vi "MAIN - PECT - Autonics.vi"() -> ()   [LabVIEW 2018]
uses:
  Control 1.ctl
  <vilib>/DAQmx/write.llb/DAQmx Write (Analog 1D Wfm NChan NSamp).vi
  <vilib>/DAQmx/read.llb/DAQmx Read (Analog 1D Wfm NChan NSamp).vi
  <vilib>/Instr/_visa.llb/VISA Configure Serial Port (Instr).vi
  <vilib>/DAQmx/create/channels.llb/DAQmx Create Channel (AI-Voltage-Basic).vi
  <vilib>/DAQmx/configure/timing.llb/DAQmx Timing (Sample Clock).vi
  <vilib>/DAQmx/configure/trigger.llb/DAQmx Start Trigger (Digital Edge).vi
  <vilib>/DAQmx/create/channels.llb/DAQmx Create Channel (AO-Voltage-Basic).vi
  <vilib>/DAQmx/miscellaneous.llb/DAQmx Fill In Error Info.vi
  Global_data.vi
  <vilib>/express/express analysis/Spectral/Block/exnSpectralBlock spectral measurements PSD poly.vi
  <vilib>/express/express analysis/Spectral/Block/exnSpectralBlock spectral measurements PSD WFM.vi
  <vilib>/express/express analysis/Spectral/XNode/ExpressSpectralMeasurementsBlockNode.xnode
  <resource>/objmgr/daqmx.rc
  <vilib>/measure/NI_MABase.lvlib
  <vilib>/Platform/NI_3dgraph.lvlib
  <vilib>/DAQmx/read.llb/DAQmx Read (Counter U32 1Chan 1Samp).vi
  <vilib>/DAQmx/create/channels.llb/DAQmx Create Channel (CI-Count Edges).vi
panel:
  out "dy":dbl[][](array[numeric])
  in  "2D Array In":dbl[][](array[numeric])
  out "Output":dbl[][](array[numeric])
  out "Current  Position (mm)":dbl=34.0
  out "Acquire":bool
  out "Numeric":dbl=34.0
  out "Enum":T1(ring)
  in  "Direction (+)":string="+"
  in  "Tab Control 3":enum32{"Control", "Data Processing"}(tab)
  in  "Home":bool
  in  "Exit":bool
  in  "Scan":bool
  in  "Move Dis(mm)":dbl=180.0
  in  "Right":bool
  in  "Forward":bool
  in  "Left":bool
  in  "Backward":bool
  in  "Stop":bool
  in  "Duty cycle %":dbl=50.0 format="%#.2f"
  in  "Pulser Trigger":tag="/Dev3/PFI0"
  in  "Edge":i32(ring)=10280 items=["Rising"=10280, "Falling"=10171]
  in  "2 Plots":bool
  in  "Offset":bool
  in  "Open csv":bool
  in  "Save Scan mode":bool caption="Save Process"
  in  "Gate 1":dbl
  in  "Gate 2":dbl=50.0
  in  "Pulse generator":T3={"Waveform Type"=2, "Amplitude"=2.0, "Frequency"=300.0} {"Frequency" format="%0.2p"; "Amplitude" format="%0.2p"; "Waveform Type" items=["Sine Wave", "Triangle Wave", "Square Wave", "Sawtooth Wave"]}
  in  "Open tdms":bool
  in  "Motor Counter Terminal":tag="PFI8"
  in  "Motor counter":tag="Dev6/ctr0"
  out "Motor Pulse Count":i32
  in  "Cursor":bool=TRUE
  in  "Repair Line Col":bool
  in  "Repair Line Row":bool
  in  "Line Col":dbl=167.0
  in  "Line Row":dbl
  in  "Y-max":dbl
  in  "Y-min":dbl
  in  "X-max":dbl
  in  "X-min":dbl
  in  "Inverse":bool caption="Scan"
  in  "ViewMode":i32(ring) items=["cwViewXYPlane", "cwViewXZPlane", "cwViewYZPlane", "cwViewUserDefined"]
  in  "Plot style":i32(ring)=5 items=["cwLine"=1, "cwPoint"=2, "cwLinePoint"=3, "cwHiddenLine"=4, "cwSurface"=5, "cwSurfaceLine"=6, "cwSurfaceNormal"=7, "cwContourLine"=8, "cwSurfaceContour"=9]
  in  "ColorMapAutoScale":bool=TRUE
  in  "Max":dbl=0.6
  in  "Min":dbl=-0.8
  in  "low cutoff freq: fl":dbl=40.0 format="%0.2f"
  in  "Filter":bool caption="Scan"
  in  "Backindex":i32
  in  "Backdata":bool caption="Scan"
  in  "Odd":bool caption="Scan"
  in  "DiffX":bool caption="Scan"
  in  "DiffY":bool caption="Scan"
  in  "Abs":bool caption="Scan"
  in  "Trim data":bool caption="Scan"
  in  "Return":bool caption="Scan"
  out "No.data":i32=160450
  in  "Tab Control 2":T4(tab)=enum."Lift-Off"
  out "Hall sensors signal":waveform(dbl)[](graph)=[{"t0"=timestamp(3764892578.4882636 s since 1904-01-01), "dt"=9.999999999999972e-06, "Y"=array[333 elements], "attributes"=variant("NI_ChannelName"=variant(string "Acquisition Task0"), "NI_UnitDescription"=variant(string "Volts"))}, {"t0"=timestamp(3764892578.4882636 s since 1904-01-01), "dt"=9.999999999999972e-06, "Y"=array[333 elements], "attributes"=variant("NI_ChannelName"=variant(string "Acquisition Task0"), "NI_UnitDescription"=variant(string "Volts"))}]
  out "Feature Extraction":dbl(graph)=2.323572486727786
  out "Power spectral density":cluster{"f0":dbl, "df":dbl, "magnitude":dbl[]}[](graph)=[{"f0"=0.0, "df"=300.30030030030116, "magnitude"=[-36.20180290677153, -20.90483721068611, -24.582468351224577, -31.42004868416134, -34.14223622321665, -37.70031787769031, -39.88091390016968, -42.570527872297575, -44.447142301932836, -46.690350484337216, -48.33027794655095, -50.25956499863859, -51.72550449795308, -53.39972065859007, -54.70440561731976, -56.21393447819807, -57.42147971089571, -58.793048346684444, -59.91128808109209, -61.1290372398805, -62.12849722306457, -63.101740591151284, -63.85083396363265, -65.0208550120241, -66.15115529173912, -67.20106472607435, -68.15468936452316, -69.13750415748885, -69.85723332409452, -70.64087441700111, -71.384683910046, -72.10421787745543, -72.7097904698358, -73.76225860074786, -74.58656508865108, -75.0441981120336, -75.64428414686775, -76.36908179290627, -76.94177220206493, -77.59120517409957, -78.33715910390706, -79.06347610630218, -79.2988856080301, -79.948424760671, -80.92068806415895, -81.77260728293177, -81.8128457263302, -84.88880957913159, -83.99592011335217, -82.99389217923485, -86.3974807070411, -83.85611495905388, -85.04739834436776, -85.25536921781624, -86.04780288701166, -86.74967696173687, -87.4250358191504, -88.33981201247339, -88.29806177830426, -88.20989281176266, -90.52050898830177, -92.73295435458243, -91.05315268517512, -89.84986904119829, -90.1243991759323, -90.08140850500105, -90.51527924221807, -91.45597364465522, -92.37045984758105, -93.05963774586344, -93.27766487428342, -92.9148468037372, -93.45821417413453, -93.416885589902, -93.97004881358691, -100.16926286158659, -103.25126222782166, -97.916857786497, -97.02995967192803, -95.41315314455832, -85.28282838125556, -91.11753429616104, -98.34800147586265, -95.8173712278324, -95.84520134535146, -96.4411910777247, -97.79095251820118, -98.76337971056503, -99.52978551104567, -99.8473172312514, -99.7267196324173, -98.48034706548019, -98.4052682848681, -98.99036338133746, -99.81336358949763, -102.0234560078495, -106.30264837390989, -114.30404783446014, -110.5666525988822, -104.07428115468332, -106.56951387813052, -113.47776650834994, -104.8106680242567, -100.96454968097595, -103.26069189712638, -101.90020017156294, -97.35968680838327, -96.96723228272809, -104.78687680019844, -114.24669922913404, -105.47220635299163, -98.95153167883362, -95.72018168888859, -96.8791317080412, -103.59986254747135, -102.32961820827316, -103.50838559146095, -106.10294185717709, -107.56586317626123, -106.21980505741361, -106.75509409282448, -105.05473267043033, -105.72146157564094, -110.05572010167114, -103.09831905065673, -100.15680582227236, -106.62655602557932, -106.04738128978546, -102.29039381337167, -107.38407353728698, -106.04045858582134, -110.27062566191805, -101.58023602789737, -100.24058473092191, -101.82465844258417, -100.49593108832102, -107.37379008605268, -111.32932544252029, -113.33511250623216, -114.1358519115806, -116.77137581473383, -119.68802410059281, -122.30038665579934, -112.78569209435597, -113.20144887694318, -114.95593587471012, -114.2945515663458, -111.45765285754484, -108.98035354159111, -102.76141277040767, -94.76605415382379, -94.53014863989041, -102.82086347018918, -104.07676059492192, -93.56502067634786, -82.01368063028869, -82.14520649644004, -92.93791399449489, -115.13858185041988, -111.90044783845615, -102.8580225326784, -106.35532255950906, -109.47985188850006, -118.27062096579498, -133.54486345969963, -117.32910571092162, -119.97301996033957]}, {"f0"=0.0, "df"=300.30030030030116, "magnitude"=[-36.20180290677153, -20.90483721068611, -24.582468351224577, -31.42004868416134, -34.14223622321665, -37.70031787769031, -39.88091390016968, -42.570527872297575, -44.447142301932836, -46.690350484337216, -48.33027794655095, -50.25956499863859, -51.72550449795308, -53.39972065859007, -54.70440561731976, -56.21393447819807, -57.42147971089571, -58.793048346684444, -59.91128808109209, -61.1290372398805, -62.12849722306457, -63.101740591151284, -63.85083396363265, -65.0208550120241, -66.15115529173912, -67.20106472607435, -68.15468936452316, -69.13750415748885, -69.85723332409452, -70.64087441700111, -71.384683910046, -72.10421787745543, -72.7097904698358, -73.76225860074786, -74.58656508865108, -75.0441981120336, -75.64428414686775, -76.36908179290627, -76.94177220206493, -77.59120517409957, -78.33715910390706, -79.06347610630218, -79.2988856080301, -79.948424760671, -80.92068806415895, -81.77260728293177, -81.8128457263302, -84.88880957913159, -83.99592011335217, -82.99389217923485, -86.3974807070411, -83.85611495905388, -85.04739834436776, -85.25536921781624, -86.04780288701166, -86.74967696173687, -87.4250358191504, -88.33981201247339, -88.29806177830426, -88.20989281176266, -90.52050898830177, -92.73295435458243, -91.05315268517512, -89.84986904119829, -90.1243991759323, -90.08140850500105, -90.51527924221807, -91.45597364465522, -92.37045984758105, -93.05963774586344, -93.27766487428342, -92.9148468037372, -93.45821417413453, -93.416885589902, -93.97004881358691, -100.16926286158659, -103.25126222782166, -97.916857786497, -97.02995967192803, -95.41315314455832, -85.28282838125556, -91.11753429616104, -98.34800147586265, -95.8173712278324, -95.84520134535146, -96.4411910777247, -97.79095251820118, -98.76337971056503, -99.52978551104567, -99.8473172312514, -99.7267196324173, -98.48034706548019, -98.4052682848681, -98.99036338133746, -99.81336358949763, -102.0234560078495, -106.30264837390989, -114.30404783446014, -110.5666525988822, -104.07428115468332, -106.56951387813052, -113.47776650834994, -104.8106680242567, -100.96454968097595, -103.26069189712638, -101.90020017156294, -97.35968680838327, -96.96723228272809, -104.78687680019844, -114.24669922913404, -105.47220635299163, -98.95153167883362, -95.72018168888859, -96.8791317080412, -103.59986254747135, -102.32961820827316, -103.50838559146095, -106.10294185717709, -107.56586317626123, -106.21980505741361, -106.75509409282448, -105.05473267043033, -105.72146157564094, -110.05572010167114, -103.09831905065673, -100.15680582227236, -106.62655602557932, -106.04738128978546, -102.29039381337167, -107.38407353728698, -106.04045858582134, -110.27062566191805, -101.58023602789737, -100.24058473092191, -101.82465844258417, -100.49593108832102, -107.37379008605268, -111.32932544252029, -113.33511250623216, -114.1358519115806, -116.77137581473383, -119.68802410059281, -122.30038665579934, -112.78569209435597, -113.20144887694318, -114.95593587471012, -114.2945515663458, -111.45765285754484, -108.98035354159111, -102.76141277040767, -94.76605415382379, -94.53014863989041, -102.82086347018918, -104.07676059492192, -93.56502067634786, -82.01368063028869, -82.14520649644004, -92.93791399449489, -115.13858185041988, -111.90044783845615, -102.8580225326784, -106.35532255950906, -109.47985188850006, -118.27062096579498, -133.54486345969963, -117.32910571092162, -119.97301996033957]}]
  in  "Add LF":bool
  in  "Save LF":bool caption="Save Process"
  in  "3D Surface":refnum<k7>(container)
  out "Record path":path=path "F:/NDT PECT/MAIN/data/0404/PECT_default.tdms" caption="selected path"
  out "Feature extraction scan":dbl[](graph)=[1.5306579414004435, 1.5317305059894941, 1.5326200461021255, 1.5328476302606462, 1.5329951898783618, 1.5347077460020615, 1.5340483037518404, 1.538225484080516, 1.5384156334587897, 1.5342859972971667, 1.5376573962153353, 1.5346896305782285, 1.5333408499151915, 1.5374363281462833, 1.5365733968770157, 1.5371060772351082, 1.5377661752425886, 1.5331402955096363, 1.5333082171292225, 1.5328402076589231, 1.5319284519372456, 1.5339877687593646, 1.5306010503955654, 1.5307758007425079, 1.5329574004689674, 1.5329084504666064, 1.5321700113481294, 1.5313764189356205, 1.5320421800954864, 1.532745648807346, 1.5335423450461179, 1.5304344707607942, 1.5310324412127772, 0.0, 0.0, 0.0, 0.0, 0.0, 0.0, 0.0, 0.0, 0.0, 0.0, 0.0, 0.0, 0.0, 0.0, 0.0, 0.0, 0.0, 0.0, 0.0, 0.0, 0.0, 0.0, 0.0, 0.0, 0.0, 0.0, 0.0, 0.0, 0.0, 0.0, 0.0, 0.0, 0.0, 0.0, 0.0, 0.0, 0.0, 0.0, 0.0, 0.0, 0.0, 0.0, 0.0, 0.0, 0.0, 0.0, 0.0, 0.0, 0.0, 0.0, 0.0, 0.0, 0.0, 0.0, 0.0, 0.0, 0.0, 0.0, 0.0, 0.0, 0.0, 0.0, 0.0, 0.0, 0.0, 0.0, 0.0, 0.0, 0.0, 0.0, 0.0, 0.0, 0.0, 0.0, 0.0, 0.0, 0.0, 0.0, 0.0, 0.0, 0.0, 0.0, 0.0, 0.0, 0.0, 0.0, 0.0, 0.0, 0.0, 0.0, 0.0, 0.0, 0.0, 0.0, 0.0, 0.0, 0.0, 0.0, 0.0, 0.0, 0.0, 0.0, 0.0, 0.0, 0.0, 0.0, 0.0]
  in  "View Mode":bool caption="Scan"
  out "Hall sensors signal lf":dbl[][](graph)
  in  "Open":bool
  in  "Filter lf":bool=TRUE caption="Scan"
  in  "Low cutoff freq: fl":dbl
  in  "Tab Control":T5(tab)=enum."          DAQ        "
  out "Start Pos X":dbl
  out "Start Pos Y":dbl
  in  "Step X":dbl=1.0
  in  "Y - length":dbl=40.0
  in  "X - length":dbl=140.0
  in  "Step Y":dbl=1.0
  in  "Multiplier":dbl=10.0
  out "Cur. Pos Y":dbl format="%#_4g"
  in  "Speed (mm/s)":dbl=10.0
  in  "Travel per Pulse (mm)":dbl=0.004
  in  "COM Y":refnum<visa-resource-name>="COM3"
  in  "COM X":refnum<visa-resource-name>="COM4"
  out "Completed":bool
  out "No. X":i32=33
  out "No. Y":i32=32
  in  "Baud Rate":u32=9600
  out "Cur. Pos X":dbl format="%#_4g"
  in  "DAQ Pulser":bool=TRUE
  in  "No. Samples":dbl=333.0
  out "Sample per Channel AO":dbl=26666.0
  in  "Pulser Cycles":i32=10
  out "Actual Sample Rate":dbl=100000.0 format="%0.2f"
  in  "Physical Channel":tag="Dev3/ai1:2"
  in  "Min Voltage":dbl=-10.0
  in  "Max Voltage":dbl=10.0
  in  "Terminal Configuration":i32(ring)=10083 items=["default"=-1, "RSE"=10083, "NRSE"=10078, "Differential"=10106, "Pseudodifferential"=12529]
  in  "Sample Clock Source 2":tag="OnboardClock"
  in  "Sample Rate":dbl=100000.0
  out "Actual Sample Rate 2":dbl=800000.0 format="%0.2f"
  in  "Physical Channel(s)":tag="Dev3/ao0:1"
  in  "Min Voltage 2":dbl=-10.0
  in  "Max Voltage 2":dbl=10.0
  in  "Sample Clock Source":tag="OnboardClock"
  in  "Sample Rate 2":dbl=800000.0 format="%#_6p"
  # "Pulse Shape"
  # "Trigger Settings"
  # "Data Processing"
  # "Time gate = %T/2"
  # "3D Surface"
  # "Process"
  # "Repair line"
  # "Hall Sensors Signal"
  # "Feature Extraction"
  # "Power Spectal Density"
  # "COM Setting"
  # "Speed Setting"
  # "Scan Setting"
  # "Pulser Channel"
  # "Pulser Timming"
  # "Sensor Channel"
  # "DAQ Timming"
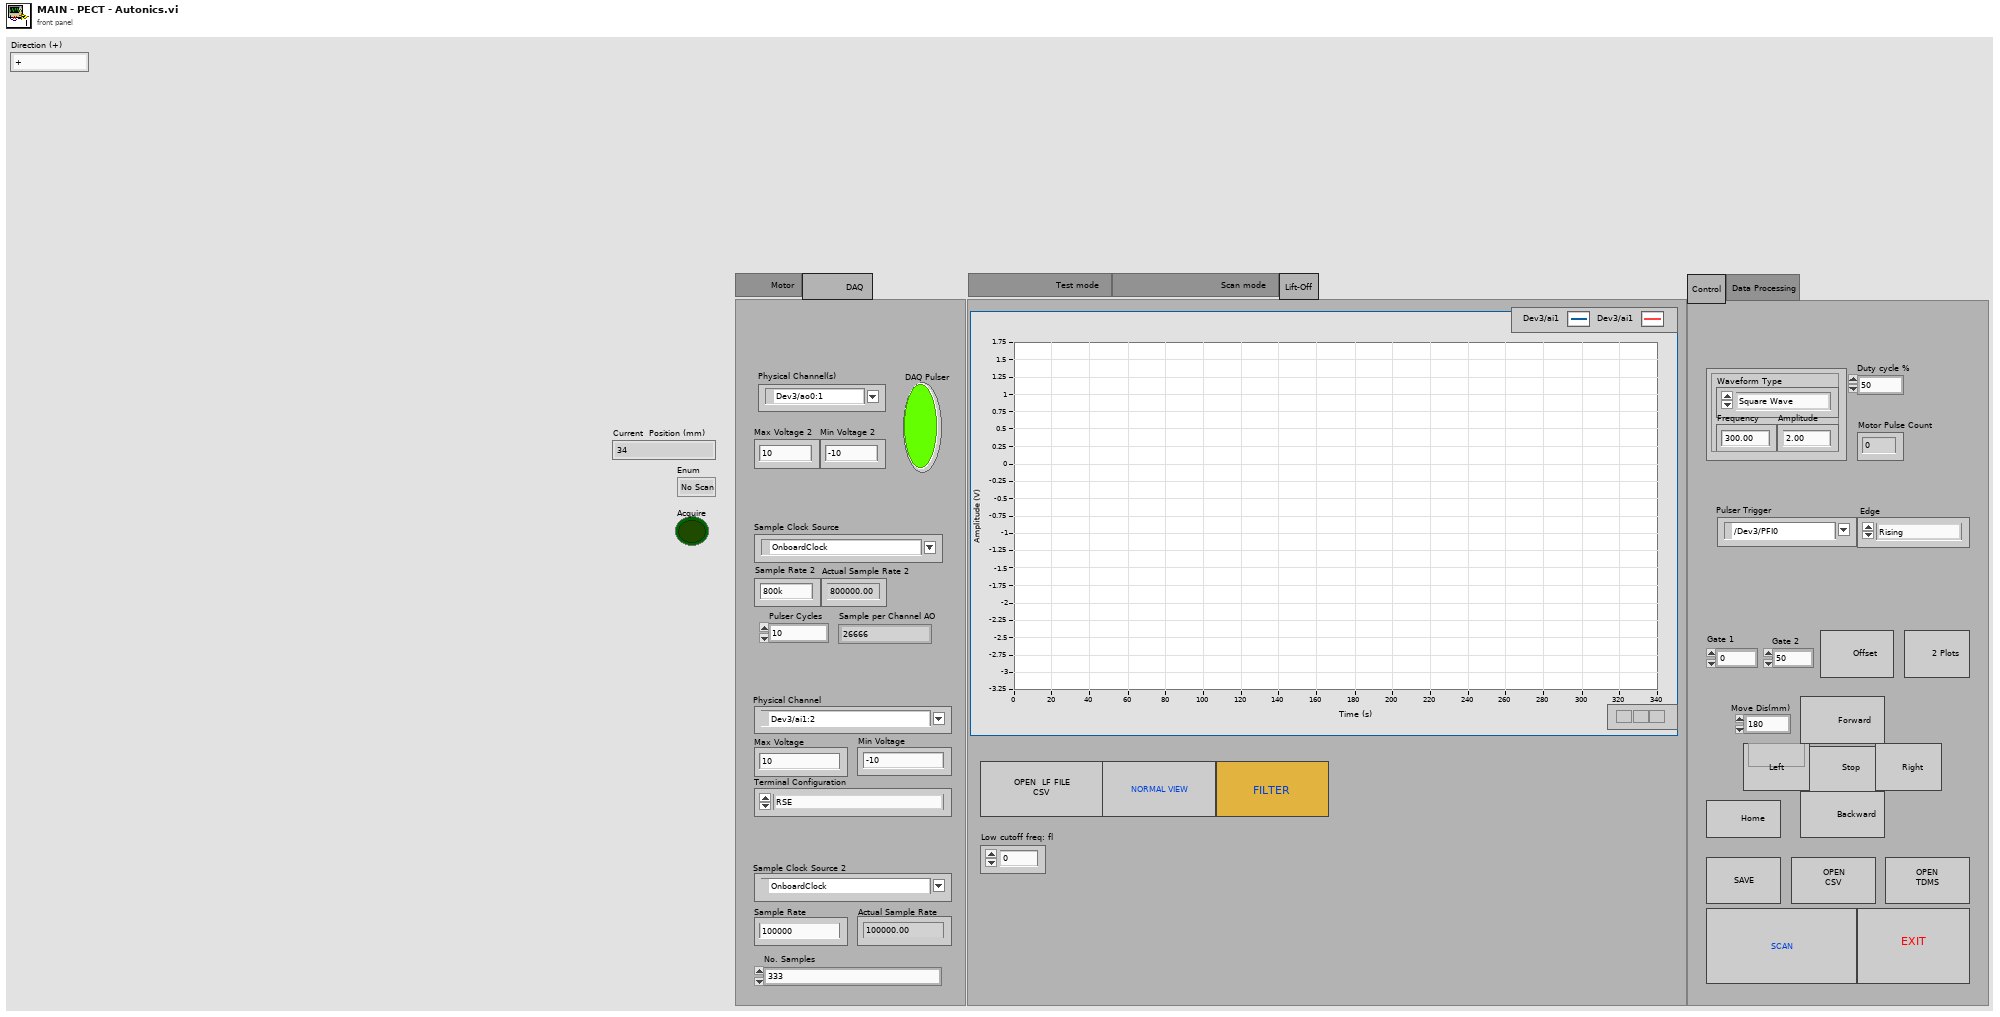
[diagram p1: front panel]
types:
  T1 = enum16{"No Scan", "Move X", "Wait X", "Move Y", "Wait Y"}
  T2 = typedef "Control 1.ctl" = dbl
  T3 = cluster{"Waveform Type":u16, "Amplitude":T2, "Frequency":dbl}
  T4 = enum32{"                    Test mode                   ", "                          Scan mode                      ", "Lift-Off"}
  T5 = enum32{"        Motor      ", "          DAQ        "}
  T6 = enum16{"open", "open or create", "create or replace", "create", "open (read-only)"}
  T7 = enum16{"Sine Wave", "Triangle Wave", "Square Wave", "Sawtooth Wave"}
  T8 = cluster{"averaging mode":u16, "weighting mode":u16, "number of averages":u32}
  T9 = cluster{"dB On (F)":bool, "unwrap phase (F)":bool, "convert to degree (F)":bool}
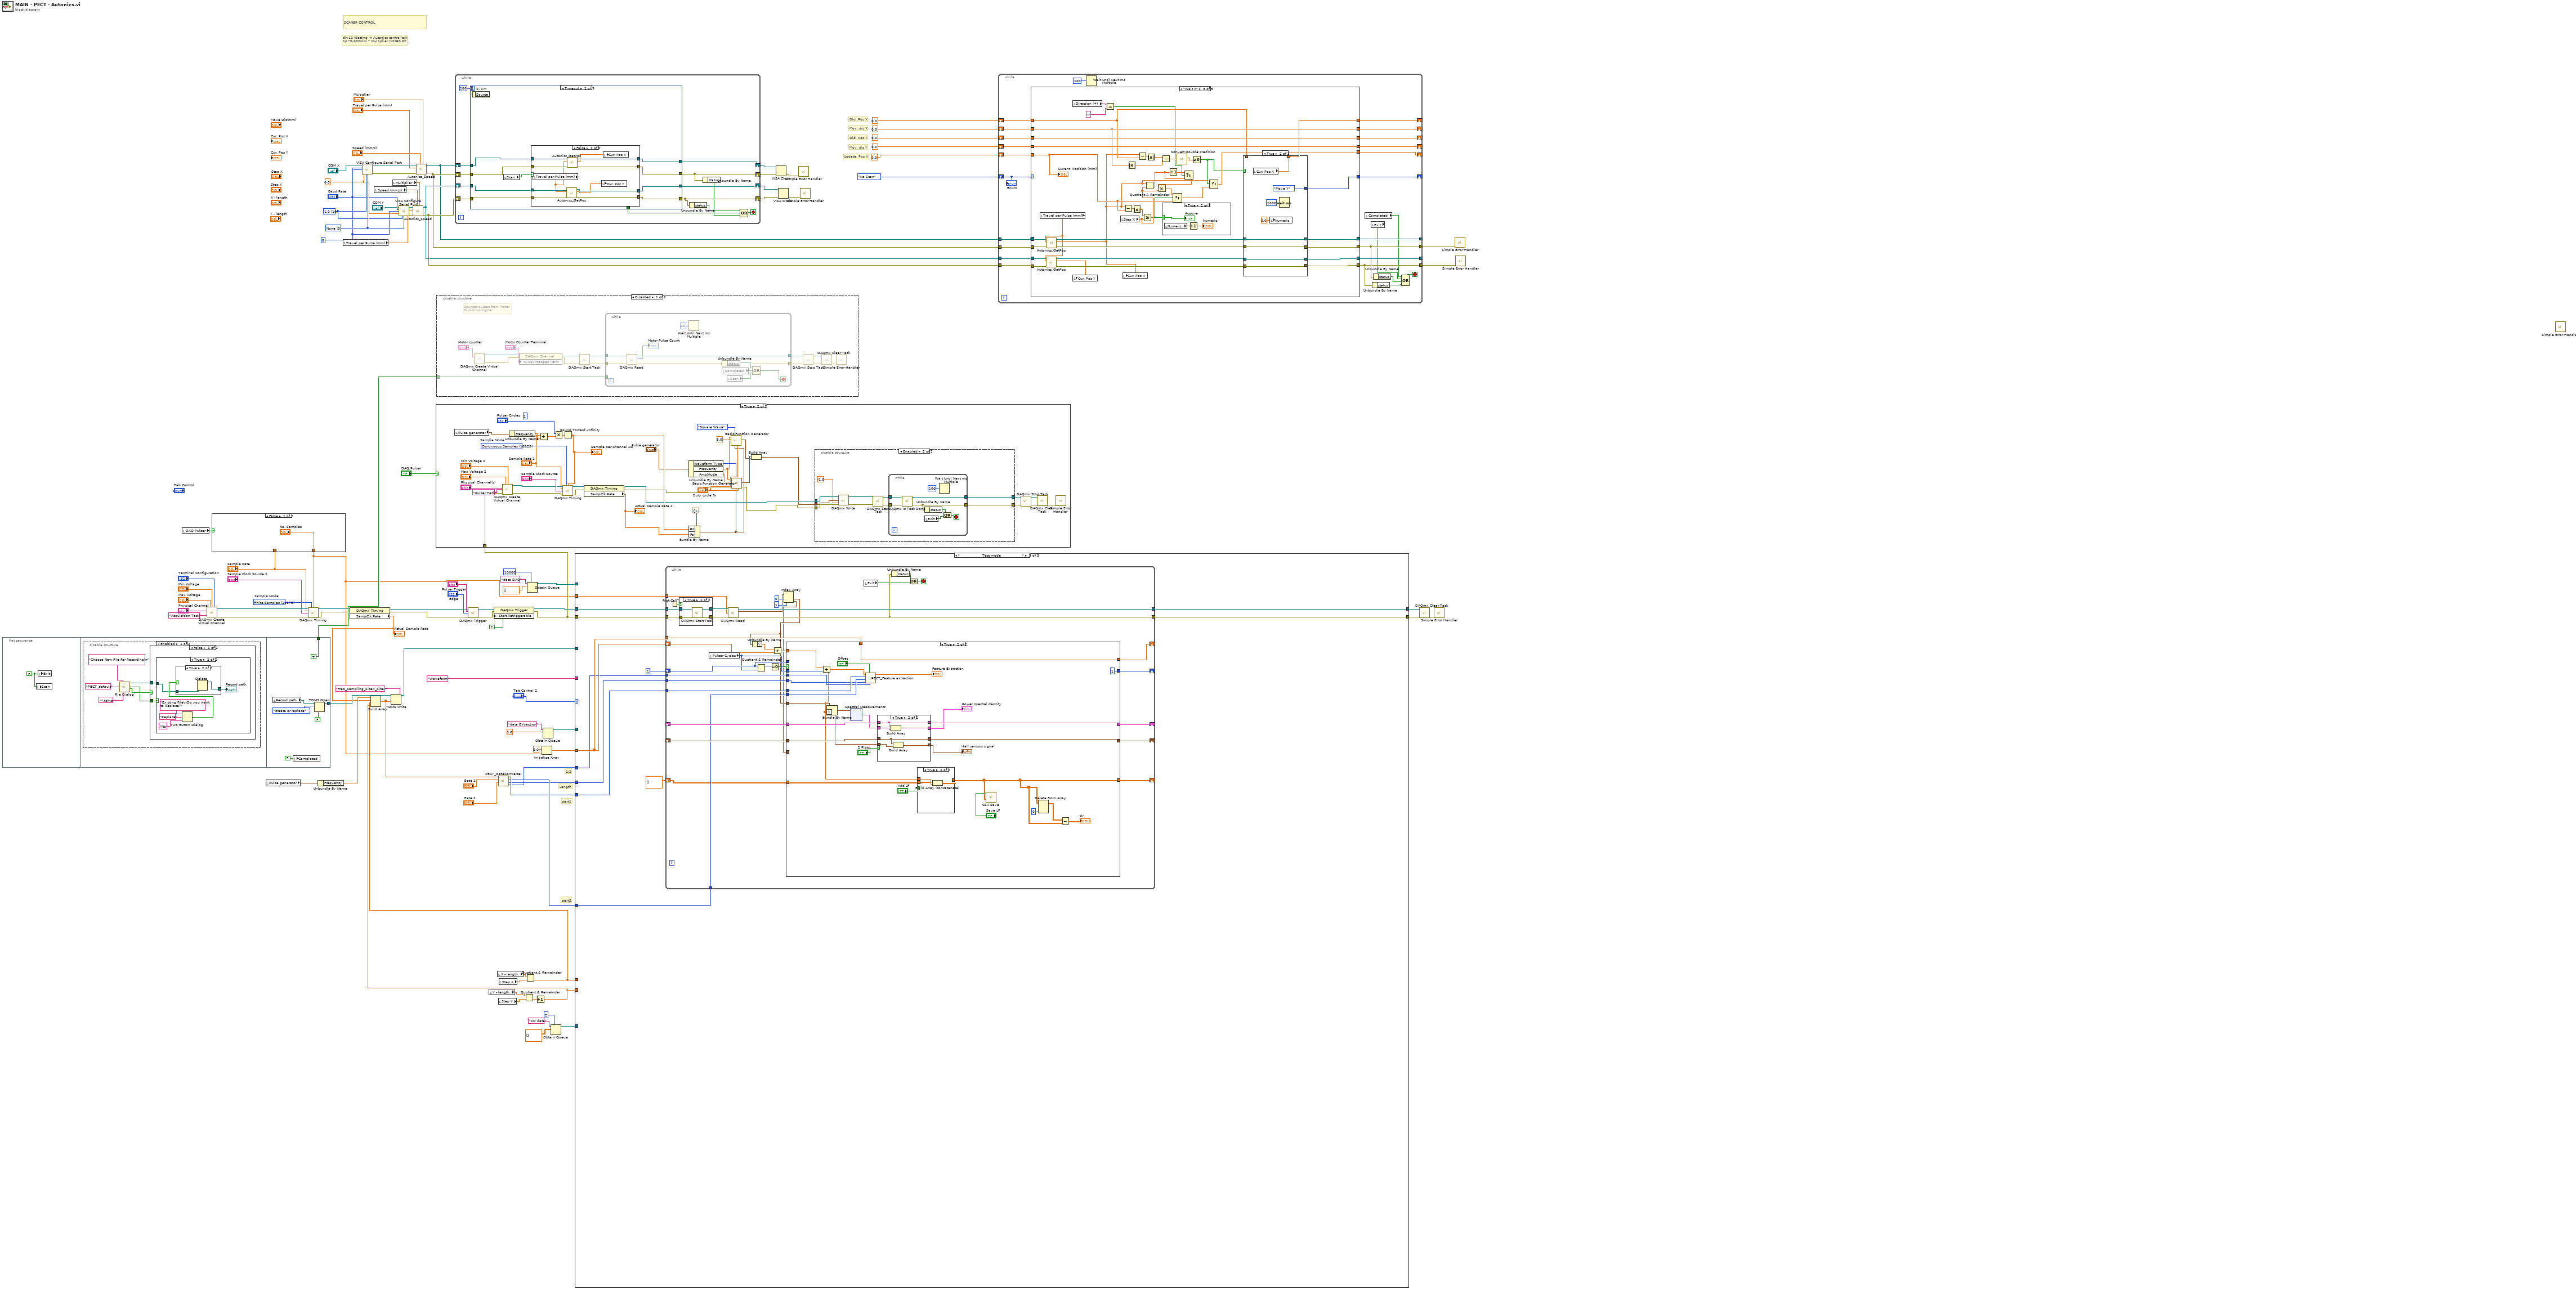
[diagram p0: block diagram]
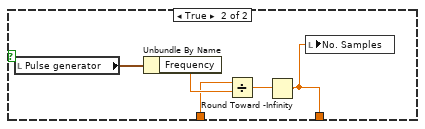
[diagram p3: hidden frame]
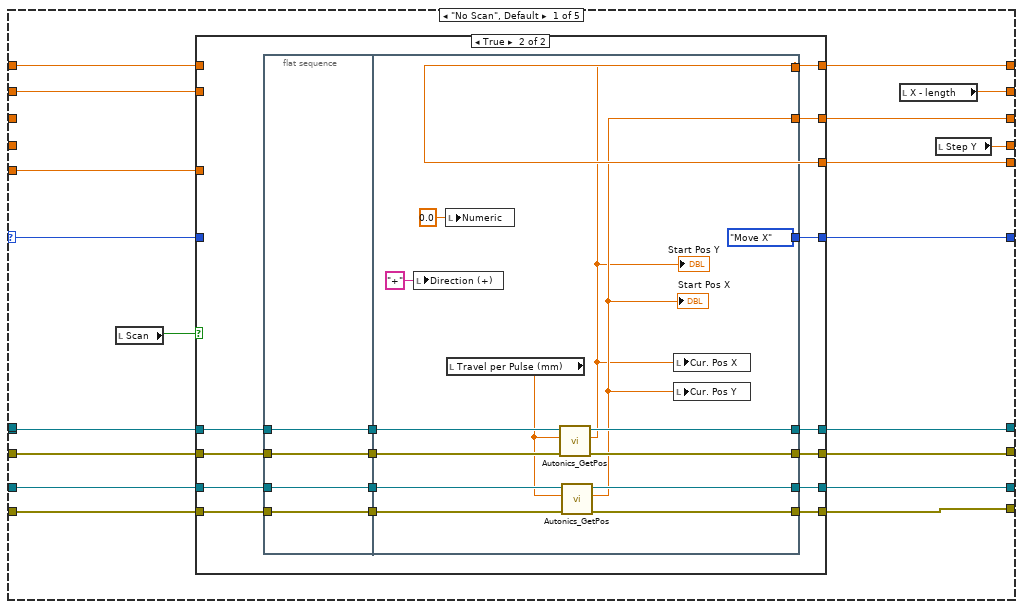
[diagram p4: hidden frame]
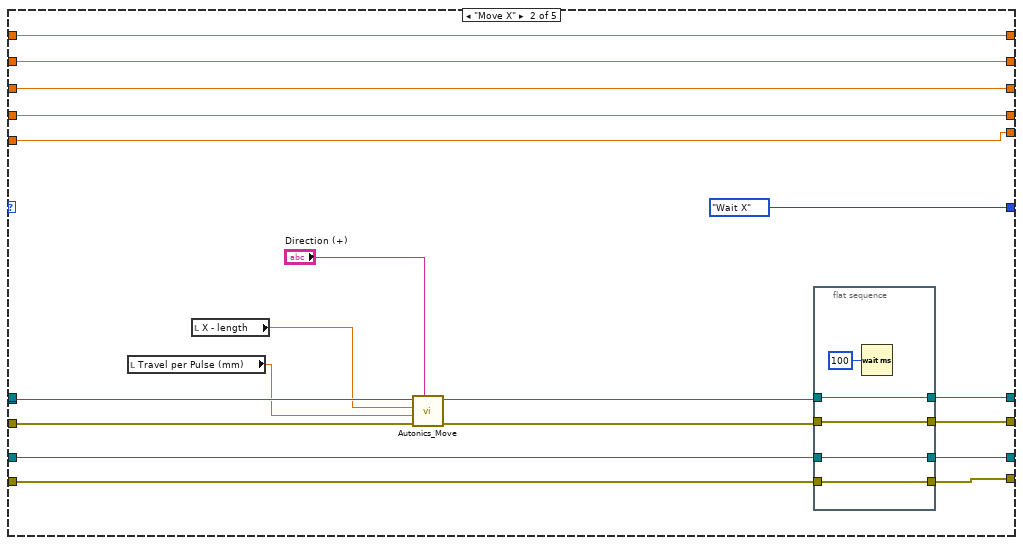
[diagram p6: hidden frame]
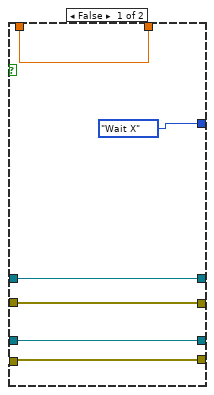
[diagram p8: hidden frame]
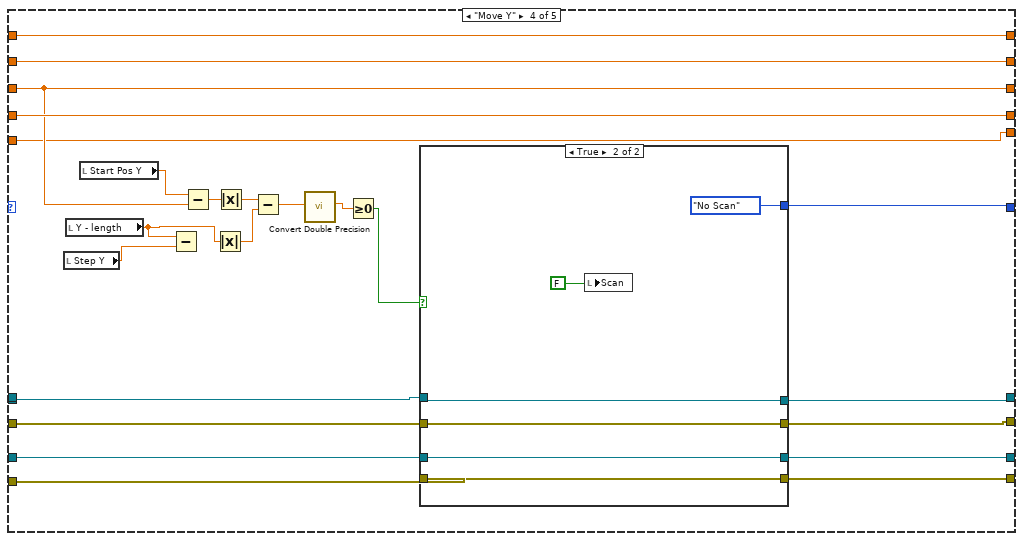
[diagram p9: hidden frame]
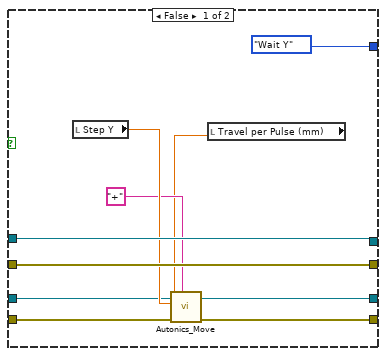
[diagram p10: hidden frame]
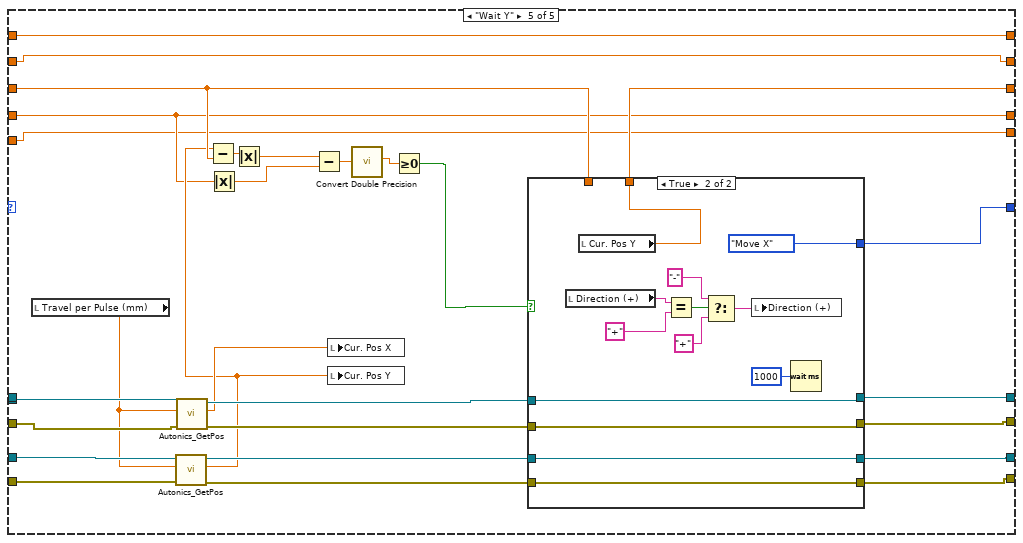
[diagram p11: hidden frame]
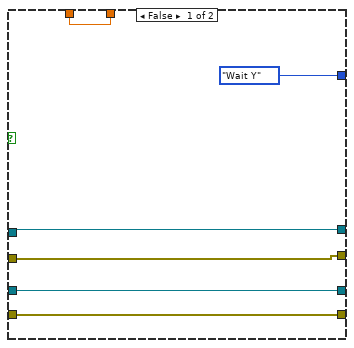
[diagram p12: hidden frame]
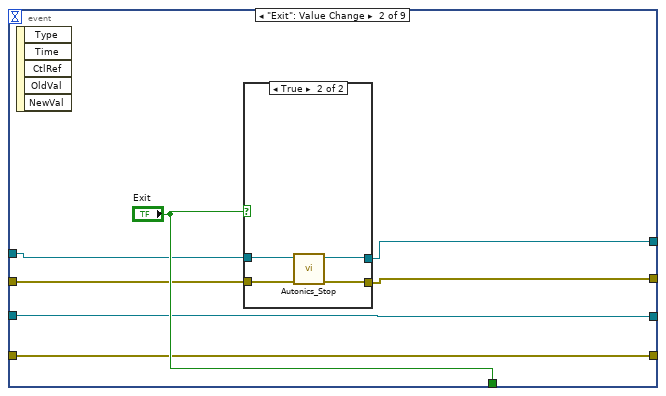
[diagram p14: hidden frame]
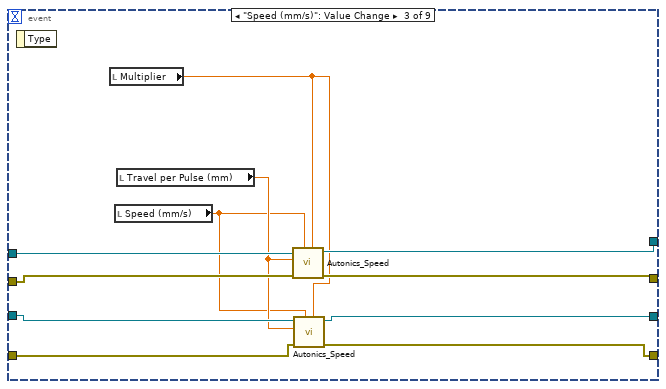
[diagram p16: hidden frame]
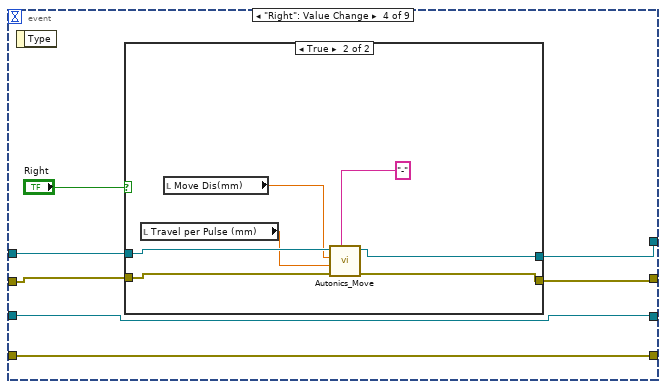
[diagram p17: hidden frame]
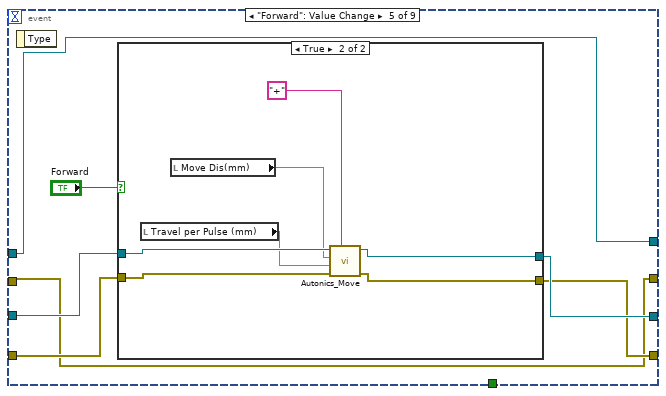
[diagram p19: hidden frame]
diagram:
  w18 = 0.0 ("Parity")
  w21 = u16 10 items=["1.0"=10, "1.5"=15, "2.0"=20] ("Stop bits")
  w22 = u16 0 items=["None", "XON/XOFF", "RTS/CTS", "XON/XOFF & RTS/CTS", "DTR/DSR", "XON/XOFF & DTR/DSR"] ("Flow control")
  w19 = u16 8 ("Data bits")
  w86 = 10178 items=["Finite Samples"=10178, "Continuous Samples"=10123, "Hardware Timed Single Point"=12522]  # Sample Mode
  # "Update. Pos X"
  # "Mov. dis Y"
  # "Old. Pos Y"
  # "Mov. dis X"
  # "Old. Pos X"
  # "div10 (Setting in Autonics controller):\n1p~0.002mm * multiplier (10)=0.02"
  # "SCANER CONTROL"
  # "1/2"
  # "start1"
  # "start2"
  # "Length"
  n1 = flat-sequence {
    tunnel: [w123] -> w66
    tunnel: [TRUE ("disable buffering (T)")] -> w46
    frame #0 {
      w99 = FALSE ("Exit")
      n2 = local write "Scan"(w99) -> ()
      n3 = local write "Exit"(w99) -> ()
    }
    frame #1 {
      n4 = disable-structure shown="Enabled" {
        frame Enabled {
          n5 = call "File Dialog"("prompt"="Choose New File For Recording\n" ("button label"), "default name"="PECT_default", "pattern (all files)"="*.tdms") -> ("selected path"=w105:path, "exists"=w101:bool, "cancelled"=w102:bool)  [unwired: 9 in, 1 out]
          n6 = case shown="False" w102 {
            tunnel: w105 -> [w106 _]
            tunnel: w101 -> [w107 _]
            frame False {
              n7 = case shown="True" w107 {
                tunnel: w106 -> [w108 w109]
                frame False {
                  n8 = local write "Record path"(w108) -> ()
                }
                frame True {
                  n9 = Two Button Dialog(message="Existing File\nDo you want to Replace?", 1:"No" ("F button name (\"Cancel\")"), 2:"Replace" ("T button name (\"OK\")")) -> (T button?=w110:bool)
                  n10 = case shown="True" w110 {
                    tunnel: w109 -> [_ w118]
                    tunnel: [path "" ("deleted path") w117] -> w111
                    frame False {
                      n11 = local write "Exit"(TRUE ("Exit")) -> ()
                    }
                    frame True {
                      n12 = Delete(path (use dialog)=w118) -> (deleted path=w117:path)  [unwired: 4 in, 2 out]
                    }
                  }
                  "Record path" <- w111
                }
              }
            }
            frame True {
              n13 = local write "Exit"(TRUE ("Exit")) -> ()
            }
          }
        }
        frame Disabled {
        }
      }
    }
    frame #2 {
      n14 = local read "Record path"() -> (w122:path)
      n15 = local write "Completed"(FALSE ("Completed")) -> ()
      n16 = TDMS Open(6:FALSE ("disable buffering (T)"), 10:T6."create or replace" ("operation"), 11:w122) -> (3:w123:refnum<k34>)  [unwired: 4 in, 1 out]
    }
  }
  n17 = local read "DAQ Pulser"() -> (w3:bool)
  n18 = call-poly <vilib>:"DAQmx Create Virtual Channel.vi"("maximum value"="Max Voltage", "minimum value"="Min Voltage", "input terminal configuration"="Terminal Configuration", "physical channels"="Physical Channel", "name to assign"="Acquisition Task") -> ("task out"=w96:refnum<k21>, "error out"=w97:errorcluster)  [unwired: 9 in]
  n19 = case shown="False" w3 {
    tunnel: ["No. Samples" w127] -> w2
    tunnel: "Sample Rate" -> [_ w129]
    frame False {
    }
    frame True {
      n20 = local read "Pulse generator"() -> (w128:T3)
      n21 = Unbundle By Name(w128) -> ("Frequency"=w131:dbl)
      n22 = Divide(x=w129, y=w131) -> (x/y=w130:dbl)
      n23 = Round Toward -Infinity(1:w130) -> (0:w127:dbl)
      n24 = local write "No. Samples"(w127) -> ()
    }
  }
  n25 = local read "Pulse generator"() -> (w54:T3)
  n26 = call-poly <vilib>:"DAQmx Timing.vi"("task/channels in"=w96, "sample mode"=w86, "samples per channel"=w2, "rate"="Sample Rate", "source"="Sample Clock Source 2", "error in"=w97) -> ("task out"=w44:refnum<k21>, "error out"=w98:errorcluster)  [unwired: 8 in]
  n27 = Unbundle By Name(w54) -> ("Frequency"=w62:dbl)
  n28 = local read "Travel per Pulse (mm)"() -> (w17:dbl)
  n29 = property class="DAQmx Timing"(reference=w44, error in=w98) -> (reference out=w42:refnum<k21>, error out=w41:errorcluster, "SampClk.Rate"=w48:dbl)
  "Actual Sample Rate" <- w48
  n30 = call-poly "VISA Configure Serial Port"("VISA resource name"="COM X", "baud rate (9600)"="Baud Rate", "data bits (8)"=w19, "parity (0:none)"=w18, "stop bits (10: 1 bit)"=w21, "flow control (0:none)"=w22) -> ("VISA resource name out"=w7:refnum<visa-resource-name>, "error out"=w8:errorcluster)  [unwired: 8 in]
  n31 = local read "Speed (mm/s)"() -> (w15:dbl)
  n32 = local read "Multiplier"() -> (w16:dbl)
  n33 = call-poly "VISA Configure Serial Port"("VISA resource name"="COM Y", "baud rate (9600)"="Baud Rate", "data bits (8)"=w19, "parity (0:none)"=w18, "stop bits (10: 1 bit)"=w21, "flow control (0:none)"=w22) -> ("VISA resource name out"=w12:refnum<visa-resource-name>, "error out"=w13:errorcluster)  [unwired: 8 in]
  n34 = call "Autonics_Speed.vi"("Multiplier"=w16, "Speed (mm/s)"=w15, "error in (no error)"=w13, "Travel per  Pulse"=w17, "VISA resource name"=w12) -> ("error out"=w26:errorcluster, "VISA resource name out"=w25:refnum<visa-resource-name>)  [unwired: 5 in]
  n35 = call "Autonics_Speed.vi"("Multiplier"="Multiplier", "Speed (mm/s)"="Speed (mm/s)", "error in (no error)"=w8, "Travel per  Pulse"="Travel per Pulse (mm)", "VISA resource name"=w7) -> ("error out"=w24:errorcluster, "VISA resource name out"=w23:refnum<visa-resource-name>)  [unwired: 5 in]
  n36 = disable-structure shown="Disabled" {
    disable-tunnel: w46 -> [w132 _]
    frame Disabled {
      # "Counter pulses from Motor\nto pick up signal"
      n37 = call-poly <vilib>:"DAQmx Create Virtual Channel.vi"("counter"="Motor counter") -> ("task out"=w139:refnum<k21>, "error out"=w141:errorcluster)  [unwired: 13 in]
      n38 = property class="DAQmx Channel"(reference=w139, error in=w141, "CI.CountEdges.Term"="Motor Counter Terminal") -> (reference out=w134:refnum<k21>, error out=w135:errorcluster)
      n39 = call <vilib>:"DAQmx Start Task.vi"("task/channels in"=w134, "error in"=w135) -> ("task out"=w136:refnum<k21>, "error out"=w133:errorcluster)  [unwired: 12 in]
      n40 = while {
        tunnel: w136 -> [w156]
        tunnel: w133 -> [w155]
        tunnel: [w147] -> w143
        tunnel: [w154] -> w142
        tunnel: [w146] -> _
        tunnel: w132 -> [w146]
        stop <- w148 stop-if-true
        n41 = call-poly <vilib>:"DAQmx Read.vi"("task/channels in"=w156, "error in"=w155) -> ("task out"=w154:refnum<k21>, "data"=→"Motor Pulse Count":u32, "error out"=w147:errorcluster)  [unwired: 11 in]
        n42 = Wait Until Next ms Multiple(millisecond multiple=u32 10 ("milliseconds to wait")) -> ()  [unwired: 1 out]
        n43 = local read "Completed"() -> (w149:bool)
        n44 = Unbundle By Name(w147) -> ("status"=w151:bool)
        n45 = local read "Scan"() -> (w150:bool)
        n46 = Compound Arithmetic op=OR(w151, w149, w150) -> (w148:bool)
      }
      n47 = call <vilib>:"DAQmx Stop Task.vi"("task/channels in"=w142, "error in"=w143) -> ("task out"=w145:refnum<k21>, "error out"=w144:errorcluster)  [unwired: 12 in]
      n48 = call <vilib>:"DAQmx Clear Task.vi"("task in"=w145, "error in"=w144) -> ("error out"=w137:errorcluster)  [unwired: 13 in]
      n49 = call <vilib>:"Simple Error Handler.vi"("error in (no error)"=w137) -> ()  [unwired: 4 in, 5 out]
    }
    frame Enabled {
    }
  }
  n50 = while {
    shift-right: [w169] -> w37
    shift-left: w23 -> [w168]
    shift-right: [w159] -> w36
    shift-left: w24 -> [w167]
    shift-right: [w162] -> w38
    shift-left: w25 -> [w164]
    shift-right: [w161] -> w39
    shift-left: w26 -> [w163]
    stop <- w166 stop-if-true
    n51 = event shown="[0] Timeout" {
      selector: _ -> [_ _ _ _ _ _ _ _ _]
      dyn-events: _ -> [_ _ _ _ _ _ _ _ _]
      timeout: 100 -> [_ _ _ _ _ _ _ _ _]
      tunnel: w168 -> [w177 w199 w217 w222 w234 w254 w267 w290 w317]
      tunnel: w167 -> [w176 w198 w216 w221 w235 w253 w266 w289 w316]
      tunnel: [w173 w197 w215 w224 w234 w256 w267 w287 w319] -> w169
      tunnel: [w172 w196 w214 w223 w235 w255 w266 w286 w318] -> w159
      tunnel: [_ "Exit" _ _ _ _ _ _ _] -> w165
      tunnel: w164 -> [w175 w194 w213 w219 w239 w251 w270 w285 w314]
      tunnel: w163 -> [w174 w195 w210 w218 w238 w250 w271 w284 w312]
      tunnel: [w171 w194 w212 w219 w237 w251 w268 w282 w313] -> w162
      tunnel: [w170 w195 w211 w218 w236 w250 w269 w283 w311] -> w161
      event Timeout {
        n52 = event-data() -> ()  [unwired: 1 in, 1 out]
        n53 = local read "Scan"() -> (w178:bool)
        n54 = case shown="False" w178 {
          tunnel: w175 -> [w189 w191]
          tunnel: w174 -> [w188 w190]
          tunnel: [w187 w191] -> w171
          tunnel: [w186 w190] -> w170
          tunnel: w176 -> [w185 w192]
          tunnel: w177 -> [w184 w193]
          tunnel: [w183 w193] -> w173
          tunnel: [w182 w192] -> w172
          frame False {
            n55 = local read "Travel per Pulse (mm)"() -> (w181:dbl)
            n56 = call "Autonics_GetPos.vi"("error in (no error)"=w188, "Travel per Pulse (mm)"=w181, "VISA resource name"=w189) -> ("error out"=w186:errorcluster, "Current  Position (mm)"=w179:dbl, "VISA resource name out"=w187:refnum<visa-resource-name>)  [unwired: 6 in]
            n57 = call "Autonics_GetPos.vi"("error in (no error)"=w185, "Travel per Pulse (mm)"=w181, "VISA resource name"=w184) -> ("error out"=w182:errorcluster, "Current  Position (mm)"=w180:dbl, "VISA resource name out"=w183:refnum<visa-resource-name>)  [unwired: 6 in]
            n58 = local write "Cur. Pos Y"(w179) -> ()
            n59 = local write "Cur. Pos X"(w180) -> ()
          }
          frame True {
          }
        }
      }
      event "Exit": Value Change {
        n60 = event-data() -> ()  [unwired: 1 in, 5 out]
        n61 = case shown="True" "Exit" {
          tunnel: [w202 w205] -> w197
          tunnel: [w201 w206] -> w196
          tunnel: w199 -> [w202 w204]
          tunnel: w198 -> [w201 w203]
          frame False {
          }
          frame True {
            n62 = call "Autonics_Stop.vi"("error in (no error)"=w203, "VISA resource name"=w204) -> ("error out"=w206:errorcluster, "VISA resource name out"=w205:refnum<visa-resource-name>)  [unwired: 8 in]
          }
        }
      }
      event "Speed (mm/s)": Value Change {
        n63 = event-data() -> ()  [unwired: 1 in, 1 out]
        n64 = local read "Multiplier"() -> (w207:dbl)
        n65 = local read "Speed (mm/s)"() -> (w208:dbl)
        n66 = local read "Travel per Pulse (mm)"() -> (w209:dbl)
        n67 = call "Autonics_Speed.vi"("Multiplier"=w207, "Speed (mm/s)"=w208, "error in (no error)"=w216, "Travel per  Pulse"=w209, "VISA resource name"=w217) -> ("error out"=w214:errorcluster, "VISA resource name out"=w215:refnum<visa-resource-name>)  [unwired: 5 in]
        n68 = call "Autonics_Speed.vi"("Multiplier"=w207, "Speed (mm/s)"=w208, "error in (no error)"=w210, "Travel per  Pulse"=w209, "VISA resource name"=w213) -> ("error out"=w211:errorcluster, "VISA resource name out"=w212:refnum<visa-resource-name>)  [unwired: 5 in]
      }
      event "Right": Value Change {
        n69 = event-data() -> ()  [unwired: 1 in, 1 out]
        n70 = case shown="True" "Right" {
          tunnel: [w225 w231] -> w224
          tunnel: [w226 w227] -> w223
          tunnel: w222 -> [w225 w233]
          tunnel: w221 -> [w226 w232]
          frame False {
          }
          frame True {
            n71 = local read "Travel per Pulse (mm)"() -> (w229:dbl)
            n72 = local read "Move Dis(mm)"() -> (w230:dbl)
            n73 = call "Autonics_Move.vi"("Direction (+)"="-", "error in (no error)"=w232, "Travel per Pulse (mm)"=w229, "Move Distance (mm)"=w230, "VISA resource name"=w233) -> ("error out"=w227:errorcluster, "VISA resource name out"=w231:refnum<visa-resource-name>)  [unwired: 5 in]
          }
        }
      }
      event "Forward": Value Change {
        n74 = event-data() -> ()  [unwired: 1 in, 1 out]
        n75 = case shown="True" "Forward" {
          tunnel: [w241 w247] -> w237
          tunnel: [w242 w246] -> w236
          tunnel: w239 -> [w241 w249]
          tunnel: w238 -> [w242 w248]
          frame False {
          }
          frame True {
            n76 = local read "Travel per Pulse (mm)"() -> (w244:dbl)
            n77 = local read "Move Dis(mm)"() -> (w245:dbl)
            n78 = call "Autonics_Move.vi"("Direction (+)"="+", "error in (no error)"=w248, "Travel per Pulse (mm)"=w244, "Move Distance (mm)"=w245, "VISA resource name"=w249) -> ("error out"=w246:errorcluster, "VISA resource name out"=w247:refnum<visa-resource-name>)  [unwired: 5 in]
          }
        }
      }
      event "Left": Value Change {
        n79 = event-data() -> ()  [unwired: 1 in, 1 out]
        n80 = case shown="True" "Left" {
          tunnel: [w258 w263] -> w256
          tunnel: [w257 w262] -> w255
          tunnel: w254 -> [w258 w265]
          tunnel: w253 -> [w257 w264]
          frame False {
          }
          frame True {
            # "Moving distance"
            n81 = local read "Travel per Pulse (mm)"() -> (w259:dbl)
            n82 = local read "Move Dis(mm)"() -> (w260:dbl)
            n83 = call "Autonics_Move.vi"("Direction (+)"="+", "error in (no error)"=w264, "Travel per Pulse (mm)"=w259, "Move Distance (mm)"=w260, "VISA resource name"=w265) -> ("error out"=w262:errorcluster, "VISA resource name out"=w263:refnum<visa-resource-name>)  [unwired: 5 in]
          }
        }
      }
      event "Backward": Value Change {
        n84 = event-data() -> ()  [unwired: 1 in, 1 out]
        n85 = case shown="True" "Backward" {
          tunnel: [w274 w279] -> w268
          tunnel: [w273 w278] -> w269
          tunnel: w270 -> [w274 w281]
          tunnel: w271 -> [w273 w280]
          frame False {
          }
          frame True {
            # "Moving distance"
            n86 = local read "Travel per Pulse (mm)"() -> (w275:dbl)
            n87 = local read "Move Dis(mm)"() -> (w276:dbl)
            n88 = call "Autonics_Move.vi"("Direction (+)"="-", "error in (no error)"=w280, "Travel per Pulse (mm)"=w275, "Move Distance (mm)"=w276, "VISA resource name"=w281) -> ("error out"=w278:errorcluster, "VISA resource name out"=w279:refnum<visa-resource-name>)  [unwired: 5 in]
          }
        }
      }
      event "Home": Value Change {
        n89 = event-data() -> ()  [unwired: 1 in, 1 out]
        n90 = case shown="True" "Home" {
          tunnel: [w294 w306] -> w287
          tunnel: [w293 w305] -> w286
          tunnel: w290 -> [w294 w310]
          tunnel: w289 -> [w293 w309]
          tunnel: w285 -> [w292 w302]
          tunnel: w284 -> [w291 w301]
          tunnel: [w292 w300] -> w282
          tunnel: [w291 w299] -> w283
          frame False {
          }
          frame True {
            n91 = call "Autonics_Home.vi"("error in (no error)"=w309, "VISA resource name"=w310) -> ("error out"=w307:errorcluster, "VISA resource name out"=w308:refnum<visa-resource-name>)  [unwired: 8 in]
            n92 = call "Autonics_Home.vi"("error in (no error)"=w301, "VISA resource name"=w302) -> ("error out"=w304:errorcluster, "VISA resource name out"=w303:refnum<visa-resource-name>)  [unwired: 8 in]
            n93 = local read "Speed (mm/s)"() -> (w297:dbl)
            n94 = local read "Travel per Pulse (mm)"() -> (w298:dbl)
            n95 = local read "Multiplier"() -> (w296:dbl)
            n96 = local write "Home"(FALSE ("Home")) -> ()
            n97 = call "Autonics_Speed.vi"("Multiplier"=w296, "Speed (mm/s)"=w297, "error in (no error)"=w307, "Travel per  Pulse"=w298, "VISA resource name"=w308) -> ("error out"=w305:errorcluster, "VISA resource name out"=w306:refnum<visa-resource-name>)  [unwired: 5 in]
            n98 = call "Autonics_Speed.vi"("Multiplier"=w296, "Speed (mm/s)"=w297, "error in (no error)"=w304, "Travel per  Pulse"=w298, "VISA resource name"=w303) -> ("error out"=w299:errorcluster, "VISA resource name out"=w300:refnum<visa-resource-name>)  [unwired: 5 in]
          }
        }
      }
      event "Stop": Value Change {
        n99 = event-data() -> ()  [unwired: 1 in, 1 out]
        n100 = case shown="False" "Stop" {
          tunnel: [w321 w328] -> w319
          tunnel: [w323 w331] -> w318
          tunnel: w317 -> [w321 w330]
          tunnel: w316 -> [w323 w329]
          tunnel: w314 -> [w322 w327]
          tunnel: [w322 w326] -> w313
          tunnel: w312 -> [w320 w325]
          tunnel: [w320 w324] -> w311
          frame False {
          }
          frame True {
            n101 = call "Autonics_Stop.vi"("error in (no error)"=w329, "VISA resource name"=w330) -> ("error out"=w331:errorcluster, "VISA resource name out"=w328:refnum<visa-resource-name>)  [unwired: 8 in]
            n102 = call "Autonics_Stop.vi"("error in (no error)"=w325, "VISA resource name"=w327) -> ("error out"=w324:errorcluster, "VISA resource name out"=w326:refnum<visa-resource-name>)  [unwired: 8 in]
          }
        }
      }
    }
    n103 = Unbundle By Name(w161) -> ("status"=w160:bool)
    n104 = Unbundle By Name(w159) -> ("status"=w158:bool)
    n105 = Compound Arithmetic op=OR(w160, w165, w158) -> (w166:bool)
  }
  n106 = call-poly <vilib>:"DAQmx Trigger.vi"("task/channels in"=w42, "source"="Pulser Trigger", "edge"="Edge", "error in"=w41) -> ("task out"=w83:refnum<k21>, "error out"=w82:errorcluster)  [unwired: 10 in]
  n107 = local read "Y - length"() -> (w5:dbl)
  n108 = property class="DAQmx Trigger"(reference=w83, error in=w82, "Start.Retriggerable"=TRUE) -> (reference out=w68:refnum<k21>, error out=w47:errorcluster)
  n109 = case shown="True" "DAQ Pulser" {
    tunnel: w47 -> [_ w370]
    frame False {
    }
    frame True {
      (unwired) 1 ("x")
      w367 = 10123 items=["Finite Samples"=10178, "Continuous Samples"=10123, "Hardware Timed Single Point"=12522]  # Sample Mode
      n110 = local read "Pulse generator"() -> (w351:T3)
      n111 = call-poly <vilib>:"DAQmx Create Virtual Channel.vi"("maximum value"="Max Voltage 2", "minimum value"="Min Voltage 2", "physical channels"="Physical Channel(s)", "name to assign"="Pulser Task", "error in"=w370) -> ("task out"=w358:refnum<k21>, "error out"=w357:errorcluster)  [unwired: 9 in]
      n112 = Unbundle By Name(w351) -> ("Frequency"=w356:dbl)
      n113 = Divide(x="Sample Rate 2", y=w356) -> (x/y=w354:dbl)
      n114 = Multiply(x="Pulser Cycles", y=w354) -> (x*y=w353:dbl)
      n115 = Round Toward -Infinity(1:w353) -> (0:w352:dbl)
      "Sample per Channel AO" <- w352
      n116 = call-poly <vilib>:"DAQmx Timing.vi"("task/channels in"=w358, "sample mode"=w367, "samples per channel"=w352, "rate"="Sample Rate 2", "source"="Sample Clock Source", "error in"=w357) -> ("task out"=w369:refnum<k21>, "error out"=w368:errorcluster)  [unwired: 8 in]
      n117 = property class="DAQmx Timing"(reference=w369, error in=w368) -> (reference out=w350:refnum<k21>, error out=w361:errorcluster, "SampClk.Rate"=w359:dbl)
      "Actual Sample Rate 2" <- w359
      n118 = Unbundle By Name("Pulse generator") -> ("Waveform Type"=w348:u16, "Frequency"=w344:dbl, "Amplitude"=w347:T2)
      n119 = Bundle By Name(cluster=cluster{"Fs":dbl, "#s":dbl} {"Fs"=1000.0, "#s"=1000.0} ("sampling info"), "#s"=w352, "Fs"=w359) -> (w338:cluster{"Fs":dbl, "#s":dbl})
      n120 = call <vilib>:"Basic Function Generator.vi"("square wave duty cycle (%)"="Duty cycle %", "sampling info"=w338, "signal type"=T7."Square Wave", "amplitude"=5.0, "frequency"=w344) -> ("signal out"=w340:waveform(dbl))  [unwired: 4 in, 2 out]
      n121 = call <vilib>:"Basic Function Generator.vi"("square wave duty cycle (%)"="Duty cycle %", "sampling info"=w338, "signal type"=w348, "error in (no error)"=w361, "amplitude"=w347, "frequency"=w344) -> ("error out"=w349:errorcluster, "signal out"=w341:waveform(dbl))  [unwired: 3 in, 1 out]
      n122 = Build Array(w341, w340) -> (w339:waveform(dbl)[])
      n123 = disable-structure shown="Enabled" {
        disable-tunnel: w339 -> [w375 w398]
        disable-tunnel: [w374 w397] -> w335
        disable-tunnel: [w373 w396] -> w332
        disable-tunnel: w350 -> [w372 w400]
        disable-tunnel: w349 -> [w371 w399]
        frame Disabled {
          n124 = while {
            tunnel: w375 -> [w386]
            shift-right: [w382] -> w374
            shift-left: w372 -> [w380]
            shift-right: [w381] -> w373
            shift-left: w371 -> [w379]
            stop <- FALSE stop-if-true
            n125 = call-poly <vilib>:"DAQmx Write.vi"("task/channels in"=w380, "data"=w386, "timeout"=-1.0, "error in"=w379) -> ("task out"=w385:refnum<k21>, "error out"=w384:errorcluster)  [unwired: 9 in, 1 out]
            n126 = call <vilib>:"DAQmx Start Task.vi"("task/channels in"=w385, "error in"=w384) -> ("task out"=w378:refnum<k21>, "error out"=w377:errorcluster)  [unwired: 12 in]
            n127 = disable-structure shown="Enabled" {
              disable-tunnel: [w392 w394] -> w382
              disable-tunnel: [w391 w393] -> w381
              disable-tunnel: w378 -> [w390 w394]
              disable-tunnel: w377 -> [w389 w393]
              frame Disabled {
                n128 = call <vilib>:"DAQmx Wait Until Done.vi"("task/channels in"=w390, "error in"=w389) -> ("task out"=w388:refnum<k21>, "error out"=w387:errorcluster)  [unwired: 12 in]
                n129 = call <vilib>:"DAQmx Stop Task.vi"("task/channels in"=w388, "error in"=w387) -> ("task out"=w392:refnum<k21>, "error out"=w391:errorcluster)  [unwired: 12 in]
              }
              frame Enabled {
              }
            }
          }
        }
        frame Enabled {
          n130 = call-poly <vilib>:"DAQmx Write.vi"("task/channels in"=w400, "data"=w398, "timeout"=-1.0, "error in"=w399) -> ("task out"=w402:refnum<k21>, "error out"=w404:errorcluster)  [unwired: 9 in, 1 out]
          n131 = call <vilib>:"DAQmx Start Task.vi"("task/channels in"=w402, "error in"=w404) -> ("task out"=w401:refnum<k21>, "error out"=w403:errorcluster)  [unwired: 12 in]
          n132 = while {
            tunnel: w401 -> [w412]
            tunnel: w403 -> [w411]
            tunnel: [w409] -> w396
            tunnel: [w410] -> w397
            stop <- w406 stop-if-true
            n133 = call <vilib>:"DAQmx Is Task Done.vi"("task/channels in"=w412, "error in"=w411) -> ("task out"=w410:refnum<k21>, "error out"=w409:errorcluster)  [unwired: 11 in, 1 out]
            n134 = Unbundle By Name(w409) -> ("status"=w407:bool)
            n135 = local read "Exit"() -> (w405:bool)
            n136 = Wait Until Next ms Multiple(millisecond multiple=u32 100) -> ()  [unwired: 1 out]
            n137 = Compound Arithmetic op=OR(w407, w405) -> (w406:bool)
          }
        }
      }
      n138 = call <vilib>:"DAQmx Stop Task.vi"("task/channels in"=w335, "error in"=w332) -> ("task out"=w334:refnum<k21>, "error out"=w333:errorcluster)  [unwired: 12 in]
      n139 = call <vilib>:"DAQmx Clear Task.vi"("task in"=w334, "error in"=w333) -> ("error out"=w366:errorcluster)  [unwired: 13 in]
      n140 = call <vilib>:"Simple Error Handler.vi"("error in (no error)"=w366) -> ()  [unwired: 4 in, 5 out]
    }
  }
  n141 = local read "X - length"() -> (w73:dbl)
  n142 = local read "Step Y"() -> (w71:dbl)
  n143 = local read "Step X"() -> (w72:dbl)
  n144 = Quotient & Remainder(x=w5, y=w71) -> (floor(x/y)=w45:dbl)  [unwired: 1 out]
  n145 = Quotient & Remainder(x=w73, y=w72) -> (floor(x/y)=w64:dbl)  [unwired: 1 out]
  n146 = Obtain Queue(max queue size (-1, unlimited)=10000, name (unnamed)="data DAQ", element data type=dbl[] [] ("data")) -> (queue out=w78:refnum<queue>)  [unwired: 2 in, 2 out]
  n147 = Increment(x=w45) -> (x+1=w4:dbl)
  n148 = Build Array(w62, w48, w64, w4) -> (w53:dbl[])
  n149 = TDMS Write(0:w66, 5:"Freq_Sampling_SizeX_SizeY" ("group name in (Untitled)"), 9:w53) -> (4:w65:refnum<k34>)  [unwired: 3 in, 3 out]
  n150 = call "PECT_GateConverse.vi"("Gate 2"="Gate 2", "Gate 1"="Gate 1", "Freq_Sampling_SizeX_SizeY"=w53) -> ("Length T/2"=w55:i32, "Length"=w56:i32, "Start 2"=w57:i32, "Start 1"=w58:i32)  [unwired: 4 in, 1 out]
  n151 = Initialize Array(0.0 ("element"), w2) -> (w79:dbl[])
  n152 = Obtain Queue(name (unnamed)="data Extraction", element data type=0.0) -> (queue out=w76:refnum<queue>)  [unwired: 3 in, 2 out]
  n153 = Obtain Queue(max queue size (-1, unlimited)=2 ("최대 큐 크기(-1,제한없음)"), name (unnamed)="2D data", element data type=dbl[][] [] ("initialized array")) -> (queue out=w50:refnum<queue>)  [unwired: 2 in, 2 out]
  n154 = case shown="\"                    Test mode                   \"" "Tab Control 2" {
    tunnel: w68 -> [w448 w696 w722]
    tunnel: [w447 w696 w721] -> w89
    tunnel: [w446 w695 w720] -> w88
    tunnel: w79 -> [w443 _ w719]
    tunnel: w47 -> [w445 w695 w718]
    tunnel: w55 -> [w444 _ w717]
    tunnel: w78 -> [w442 _ _]
    tunnel: w76 -> [w421 _ _]
    tunnel: w64 -> [w416 _ _]
    tunnel: w4 -> [w417 _ _]
    tunnel: w56 -> [w429 _ w715]
    tunnel: w58 -> [w428 _ w714]
    tunnel: w57 -> [w427 _ w713]
    tunnel: w65 -> [w426 _ _]
    tunnel: "Waveform" ("group name in (Untitled)") -> [w423 _ _]
    tunnel: w50 -> [w418 _ _]
    tunnel: w2 -> [w413 _ w712]
    frame "                          Scan mode                      ", Default {
      # "Column"
      # "Row"
      n155 = Initialize Array(0.0 ("element"), w416, w417) -> (w435:dbl[][])
      n156 = local read "3D Surface"() -> (w430:refnum<k7>)
      n157 = Matrix Size(0:w435) -> (1:w436:i32, 2:w437:i32)
      n158 = Decrement(x=w436) -> (x-1=w440:i32)
      n159 = Decrement(x=w437) -> (x-1=w439:i32)
      n160 = call "Surface_AxesScale.vi"("Y-axis Max"=w439, "X-axis max"=w440, "3D Surface"=w430, "Auto Scale"=FALSE) -> ()  [unwired: 8 in]
      n161 = while {
        shift-right: [w494] -> _
        shift-left: 0 -> [w496]
        shift-right: [w493] -> _
        shift-left: 0 -> [w495]
        tunnel: w421 -> [w492]
        shift-right: [w484] -> w414
        shift-left: w435 -> [w491]
        shift-right: [w487] -> _
        shift-left: TRUE ("Output Direction") -> [w488]
        tunnel: w418 -> [w486]
        tunnel: [w485] -> w419
        stop <- w489 stop-if-true
        n162 = local read "Scan"() -> (w483:bool)
        n163 = local read "Completed"() -> (w482:bool)
        n164 = Compound Arithmetic op=AND(invert w483, invert w482) -> (w481:bool)
        n165 = case shown="False" w481 {
          tunnel: w496 -> [w513 w559]
          tunnel: w495 -> [w512 w558]
          tunnel: [w511 w559] -> w494
          tunnel: [w505 w558] -> w493
          tunnel: w492 -> [w510 w551]
          tunnel: w491 -> [w509 w555]
          tunnel: [w502 w538] -> w484
          tunnel: [w508 _] -> w480
          tunnel: w488 -> [w507 w557]
          tunnel: [w506 w557] -> w487
          tunnel: w486 -> [w503 w540]
          tunnel: [w501 w551] -> w485
          frame False {
            n166 = Dequeue Element(queue=w510, timeout in ms (-1)=5000) -> (queue out=w501:refnum<queue>, element=w504:dbl)  [unwired: 1 in, 2 out]
            n167 = call "EletoMatr_1channel.vi"("Input Array X"=w509, "Input data"=w504, "In Row"=w513, "In Column"=w512, "Input Direction"=w507) -> ("Completed"=w508:bool, "Out Array X"=w502:dbl[][], "Out Row"=w511:i32, "Output Direction"=w506:bool, "Out Column"=w505:i32)  [unwired: 6 in]
            n168 = Lossy Enqueue Element(queue=w503, element=w502) -> ()  [unwired: 1 in, 4 out]
          }
          frame True {
            n169 = local read "Gate 1"() -> (w554:dbl)
            n170 = local read "Gate 2"() -> (w553:dbl)
            n171 = Wait Until Next ms Multiple(millisecond multiple=u32 100 ("ms 배수")) -> ()  [unwired: 1 out]
            n172 = local read "Offset"() -> (w545:bool)
            n173 = call "TDMS_Open.vi"("Offset"=w545, "Gate 2"=w553, "Gate 1"=w554, "Input 2D"=w555, "Open"="Open tdms") -> ("Output 2D"=w518:dbl[][])  [unwired: 5 in, 1 out]
            n174 = case shown="True" "Open tdms" {
              tunnel: w518 -> [_ w560]
              frame False {
              }
              frame True {
                n175 = global write "Global_data.vi" "global 2d graph"(w560) -> ()
              }
            }
            n176 = call "RepairLine.vi"("Repair Line Col"="Repair Line Col", "Repair Line Row"="Repair Line Row", "Line Col"="Line Col", "Line Row"="Line Row", "Array In"=w518) -> ("Array Repaired"=w532:dbl[][])  [unwired: 6 in]
            n177 = call "CSV Open.vi"("2D Array In"=w532, "Open"="Open csv") -> ("2D Array Out"=w539:dbl[][])  [unwired: 9 in]
            n178 = call "Backdata.vi"("Backindex"="Backindex", "Array in"=w539, "Backdata"="Backdata") -> ("Array out"=w521:dbl[][])
            n179 = call "TrimXY.vi"("X-max"="Y-max", "X-min"="Y-min", "Y-max"="X-max", "Y-min"="X-min", "Array In"=w521, "Trim data"="Trim data") -> ("Array Trim Out"=w520:dbl[][])  [unwired: 5 in]
            n180 = global read "Global_data.vi" "global 2d graph"() -> (w515:dbl[][])
            n181 = call "Inverse.vi"(10:"Inverse"=w520, 11:"Inverse"="Inverse") -> ("Array out"=w516:dbl[][])  [unwired: 9 in]
            n182 = call "Return data.vi"("Array Return"=w515, "Array Input"=w516, "Return"="Return") -> ("Array out"=w514:dbl[][])  [unwired: 8 in]
            n183 = call "Abs.vi"("Input"=w514, "Abs"="Abs") -> ("Array out"=w544:dbl[][])  [unwired: 9 in]
            n184 = call "DiffX.vi"("Array in"=w544, "DiffX"="DiffX") -> ("Array out"=w549:dbl[][])  [unwired: 1 in]
            n185 = call "DiffY.vi"("Array in"=w549, "DiffY"="DiffY") -> ("Array out"=w547:dbl[][])  [unwired: 1 in]
            n186 = call "Odd.vi"("Odd"="Odd", "Array In"=w547) -> ("Array Out"=w536:dbl[][])  [unwired: 9 in]
            n187 = call "Filter_Lowpass - 2D.vi"("Filter"="Filter", "Input 2D"=w536, "low cutoff freq: fl"="low cutoff freq: fl") -> ("Output"=w535:dbl[][])  [unwired: 6 in]
            n188 = case shown="True" TRUE {
              tunnel: w535 -> [w561 w562]
              tunnel: [w561 w562] -> w538
              tunnel: w540 -> [_ w563]
              frame False {
              }
              frame True {
                n189 = local read "3D Surface"() -> (w567:refnum<k7>)
                n190 = Matrix Size(0:w562) -> (1:w568:i32, 2:w565:i32)
                n191 = Decrement(x=w568) -> (x-1=w566:i32)
                n192 = Decrement(x=w565) -> (x-1=w564:i32)
                n193 = call "Surface_AxesScale.vi"("Y-axis Max"=w564, "X-axis max"=w566, "3D Surface"=w567, "Auto Scale"=FALSE) -> ()  [unwired: 8 in]
                n194 = Lossy Enqueue Element(queue=w563, element=w562) -> ()  [unwired: 1 in, 4 out]
              }
            }
          }
        }
        "Output" <- w484
        n195 = case shown="True" w480 {
          selector: w480 -> [w497 w498]
          tunnel: [w497 w498] -> w479
          frame False {
          }
          frame True {
            n196 = Wait (ms)(milliseconds to wait=u32 200) -> ()  [unwired: 1 out]
          }
        }
        "Completed" <- w479
        n197 = local read "Exit"() -> (w490:bool)
        n198 = Compound Arithmetic op=OR(w479, w490) -> (w489:bool)
        "No. Y" <- w495
        "No. X" <- w496
      }
      n199 = while {
        tunnel: w448 -> [w579]
        tunnel: [w578] -> w447
        tunnel: [w577] -> w446
        tunnel: w445 -> [w576]
        tunnel: w442 -> [w575]
        tunnel: w413 -> [w570]
        stop <- w571 stop-if-true
        n200 = case shown="True" "Scan" {
          tunnel: w579 -> [w581 w587]
          tunnel: [w581 w586] -> w578
          tunnel: [w580 w585] -> w577
          tunnel: w576 -> [w580 w584]
          tunnel: w575 -> [_ w583]
          tunnel: w570 -> [_ w582]
          frame False {
          }
          frame True {
            n201 = while {
              tunnel: w587 -> [w601]
              tunnel: [w604] -> w586
              tunnel: [w603] -> w585
              tunnel: w584 -> [w600]
              tunnel: w583 -> [w602]
              tunnel: w582 -> [w592]
              stop <- w593 stop-if-true
              n202 = First Call?() -> (First Call?: T/F=w597:bool)
              n203 = case shown="True" w597 {
                tunnel: w601 -> [w605 w610]
                tunnel: w600 -> [w606 w609]
                tunnel: [w605 w608] -> w599
                tunnel: [w606 w607] -> w598
                frame False {
                }
                frame True {
                  n204 = call <vilib>:"DAQmx Start Task.vi"("task/channels in"=w610, "error in"=w609) -> ("task out"=w608:refnum<k21>, "error out"=w607:errorcluster)  [unwired: 12 in]
                }
              }
              n205 = call-poly <vilib>:"DAQmx Read.vi"("task/channels in"=w599, "timeout"=w592, "error in"=w598) -> ("task out"=w604:refnum<k21>, "data"=w590:waveform(dbl)[], "error out"=w603:errorcluster)  [unwired: 10 in]
              n206 = Index Array(array=w590, index=0 ("index (row)")) -> (element=w589:waveform(dbl))
              n207 = Unbundle By Name(w589) -> ("Y"=w588:dbl[])
              n208 = Enqueue Element(queue=w602, element=w588) -> ()  [unwired: 2 in, 3 out]
              n209 = Unbundle By Name(w603) -> ("status"=w594:bool)
              n210 = local read "Completed"() -> (w596:bool)
              n211 = local read "Exit"() -> (w595:bool)
              n212 = Compound Arithmetic op=OR(w594, w596, w595) -> (w593:bool)
            }
          }
        }
        n213 = local read "Completed"() -> (w572:bool)
        n214 = local read "Exit"() -> (w573:bool)
        n215 = Compound Arithmetic op=OR(w572, w573) -> (w571:bool)
      }
      n216 = while {
        shift-right: [w627] -> _
        shift-left: w443 -> [w631]
        tunnel: w443 -> [w630]
        tunnel: w444 -> [w629]
        tunnel: w442 -> [w628]
        tunnel: w421 -> [w626]
        shift-right: [w623] -> _
        shift-left: 0 -> [w624]
        tunnel: w429 -> [w622]
        tunnel: w428 -> [w621]
        tunnel: w427 -> [w620]
        tunnel: w426 -> [w619]
        tunnel: [w618] -> w425
        tunnel: [w617] -> w424
        tunnel: w423 -> [w616]
        shift-right: [w614] -> _
        shift-left: 0 -> [w615]
        stop <- w611 stop-if-true
        n217 = local read "Scan"() -> (w625:bool)
        n218 = case shown="True" w625 {
          tunnel: w631 -> [w636 w649]
          tunnel: w630 -> [_ w655]
          tunnel: w629 -> [_ w654]
          tunnel: w628 -> [_ w653]
          tunnel: [w636 w652] -> w627
          tunnel: w626 -> [_ w651]
          tunnel: w624 -> [w635 w647]
          tunnel: [w635 w646] -> w623
          tunnel: w622 -> [_ w645]
          tunnel: w621 -> [_ w644]
          tunnel: w620 -> [_ w643]
          tunnel: w619 -> [w633 w642]
          tunnel: [w633 w641] -> w618
          tunnel: [_ w640] -> w617
          tunnel: w616 -> [_ w639]
          tunnel: w615 -> [w632 w638]
          tunnel: [w632 w637] -> w614
          frame False {
            n219 = Wait Until Next ms Multiple(millisecond multiple=u32 100 ("ms 배수")) -> ()  [unwired: 1 out]
          }
          frame True {
            n220 = local read "Pulser Cycles"() -> (w648:i32)
            n221 = Increment(x=w647) -> (x+1=w646:i32)
            n222 = Dequeue Element(queue=w653) -> (element=w650:dbl[])  [unwired: 2 in, 3 out]
            n223 = Quotient & Remainder(x=w646, y=w648) -> (x-y*floor(x/y)=w656:i32)  [unwired: 1 out]
            n224 = Add(x=w650, y=w649) -> (x+y=w658:dbl[])
            n225 = Equal To 0?(x=w656) -> (x = 0?=w657:bool)
            n226 = case shown="True" w657 {
              tunnel: w648 -> [_ w679]
              tunnel: w658 -> [w661 w677]
              tunnel: [w661 w680] -> w652
              tunnel: w655 -> [_ w680]
              tunnel: w654 -> [_ w673]
              tunnel: w651 -> [_ w678]
              tunnel: w645 -> [_ w674]
              tunnel: w644 -> [_ w676]
              tunnel: w643 -> [_ w675]
              tunnel: w642 -> [w660 w667]
              tunnel: [w660 w665] -> w641
              tunnel: [_ w664] -> w640
              tunnel: w639 -> [_ w666]
              tunnel: w638 -> [w659 w669]
              tunnel: [w659 w668] -> w637
              frame False {
                n227 = disable-structure shown="비활성화" {
                  frame Disabled {
                    n228 = Wait Until Next ms Multiple(millisecond multiple=u32 100 ("ms 배수")) -> ()  [unwired: 1 out]
                  }
                  frame Enabled {
                  }
                }
              }
              frame True {
                n229 = Divide(x=w677, y=w679) -> (x/y=w663:dbl[])
                n230 = local read "Offset"() -> (w672:bool)
                n231 = disable-structure shown="Enabled" {
                  disable-tunnel: [w683 w684] -> w670
                  disable-tunnel: w669 -> [w682 _]
                  disable-tunnel: [w681 _] -> w668
                  frame Disabled {
                    n232 = local read "Motor Pulse Count"() -> (w681:i32)
                    n233 = Not Equal?(x=w681, y=w682) -> (x != y?=w683:bool)
                  }
                  frame Enabled {
                    n234 = local read "Acquire"() -> (w684:bool)
                  }
                }
                n235 = call "PECT_Feature extraction.vi"("Length T/2"=w673, "Offset"=w672, "Length"=w674, "Start 2"=w675, "Start 1"=w676, "Pulse signal in"=w663) -> ("Feature extraction out"=w671:dbl)  [unwired: 5 in]
                n236 = case shown="True" w670 {
                  tunnel: w678 -> [_ w693]
                  tunnel: w671 -> [_ w692]
                  tunnel: w667 -> [w685 w691]
                  tunnel: w666 -> [_ w690]
                  tunnel: w663 -> [_ w686]
                  tunnel: [w685 w689] -> w665
                  tunnel: [_ w688] -> w664
                  frame False {
                  }
                  frame True {
                    n237 = TDMS Write(0:w691, 5:w690, 9:w686) -> (4:w689:refnum<k34>, 15:w688:errorcluster)  [unwired: 3 in, 2 out]
                    n238 = Enqueue Element(queue=w693, element=w692) -> ()  [unwired: 2 in, 3 out]
                    n239 = local write "Acquire"(FALSE ("Acquire")) -> ()
                  }
                }
              }
            }
          }
        }
        n240 = local read "Completed"() -> (w613:bool)
        n241 = local read "Exit"() -> (w612:bool)
        n242 = Compound Arithmetic op=OR(w613, w612) -> (w611:bool)
        "No.data" <- w624
      }
      n243 = while {
        tunnel: w418 -> [w476]
        tunnel: w417 -> [_]
        tunnel: w416 -> [_]
        tunnel: [w473] -> w415
        stop <- w474 stop-if-true
        n244 = local read "Output"() -> (w464:dbl[][])
        n245 = local read "No. Y"() -> (w471:i32)
        n246 = call "CursorPosition.vi"("Cursor No."=1.0, "Cursor"="Cursor", "3D Surface Analysis"="3D Surface") -> ("Cursor Y"=w466:dbl)  [unwired: 6 in, 2 out]
        n247 = Dequeue Element(queue=w476, timeout in ms (-1)=3000) -> (queue out=w473:refnum<queue>)  [unwired: 1 in, 3 out]
        n248 = Add(x=w471, y=w466) -> (x+y=w470:dbl)
        n249 = Index Array(array=w464, index (col)=w470) -> (element=→"Feature extraction scan":dbl[])  [unwired: 1 in]
        n250 = call <vilib>:"3D Surface.vi"("z matrix"=w464, "3D graph"="3D Surface") -> ()  [unwired: 8 in, 2 out]
        n251 = local read "Completed"() -> (w472:bool)
        n252 = local read "Exit"() -> (w475:bool)
        n253 = Compound Arithmetic op=OR(w472, w475) -> (w474:bool)
        n254 = Wait Until Next ms Multiple(millisecond multiple=u32 100 ("ms 배수")) -> ()  [unwired: 1 out]
      }
      n255 = Release Queue(queue=w415) -> ()  [unwired: 2 in, 3 out]
      n256 = while {
        stop <- w449 stop-if-true
        n257 = event shown="[0] \"Plot style\", \"ViewMode\": Value Change" {
          selector: _ -> [_ _ _]
          dyn-events: _ -> [_ _ _]
          timeout: _ -> [_ _ _]
          tunnel: [_ w453 _] -> w449
          event "Plot style", "ViewMode": Value Change {
            n258 = event-data() -> ()  [unwired: 1 in, 2 out]
            n259 = local read "3D Surface"() -> (w452:refnum<k7>)
            n260 = property class="CWGraph3D"(reference=w452, "ViewMode"="ViewMode") -> ()  [unwired: 1 in, 2 out]
            n261 = call <vilib>:"Basic Properties.vi"("3D graph"=w452, "plot style"="Plot style") -> ()  [unwired: 12 in, 2 out]
          }
          event "Exit": Value Change {
            n262 = event-data() -> ()  [unwired: 1 in, 1 out]
            n263 = local read "Exit"() -> (w453:bool)
          }
          event "Max", "Min", "ColorMapAutoScale": Value Change {
            n264 = event-data() -> ()  [unwired: 1 in, 5 out]
            n265 = local read "3D Surface"() -> (w454:refnum<k7>)
            n266 = call "Surface_ColorScale.vi"("ColorMapAutoScale"="ColorMapAutoScale", "Min"="Min", "Max"="Max", "3D Surface_"=w454) -> ("Min 2"=w458:dbl, "Max 2"=w457:dbl)  [unwired: 1 in, 2 out]
            n267 = local write "Max"(w457) -> ()
            n268 = local write "Min"(w458) -> ()
          }
        }
      }
      n269 = TDMS Close(8:w424, 11:w425) -> (0:w422:errorcluster)  [unwired: 1 out]
      n270 = call <vilib>:"Simple Error Handler.vi"("error in (no error)"=w422) -> ()  [unwired: 2 in, 7 out]
      n271 = Release Queue(queue=w419) -> ()  [unwired: 2 in, 3 out]
      n272 = while {
        tunnel: w414 -> [w462]
        stop <- w461 stop-if-true
        n273 = call "CSV Save.vi"("Array"=w462, "Save Button"="Save Scan mode") -> ()  [unwired: 9 in, 1 out]
        n274 = Wait Until Next ms Multiple(millisecond multiple=u32 100 ("ms 배수")) -> ()  [unwired: 1 out]
        n275 = local read "Exit"() -> (w461:bool)
      }
    }
    frame "Lift-Off" {
      n276 = while {
        shift-right: [w705] -> _
        shift-left: "2D Array In" -> [w706]
        stop <- w710 stop-if-true
        n277 = call "CSV Open.vi"("2D Array In"=w706, "Open"="Open") -> ("2D Array Out"=w705:dbl[][])  [unwired: 9 in]
        n278 = Delete From Array(array=w705, index (col)=0 ("disabled index (col)")) -> (array with subset deleted=w707:dbl[][])  [unwired: 2 in, 1 out]
        n279 = Subtract(x=w707, y=w705) -> (x-y=w703:dbl[][])
        n280 = Transpose 2D Array(2D array=w703) -> (transposed array=w700:dbl[][])
        n281 = call "Filter_Lowpass - 2D.vi"("Filter"="Filter lf", "Input 2D"=w700, "low cutoff freq: fl"="Low cutoff freq: fl") -> ("Output"=w702:dbl[][])  [unwired: 6 in]
        n282 = Transpose 2D Array(2D array=w702) -> (transposed array=w699:dbl[][])
        n283 = Select(t=w699, s="View Mode", f=w705) -> (s? t:f=→"Hall sensors signal lf":dbl[][])
        n284 = local read "Exit"() -> (w710:bool)
      }
    }
    frame "                    Test mode                   " {
      n285 = while {
        tunnel: w722 -> [w739]
        tunnel: w718 -> [w738]
        tunnel: [w756] -> w720
        tunnel: [w757] -> w721
        shift-right: [w752] -> _
        shift-left: w719 -> [w753]
        tunnel: w719 -> [w751]
        shift-right: [w749] -> _
        shift-left: _ -> [w748]
        tunnel: w717 -> [w747]
        shift-right: [w746] -> _
        shift-left: _ -> [w745]
        shift-right: [w743] -> _
        shift-left: 1 ("Average") -> [w742]
        tunnel: w715 -> [w735]
        tunnel: w714 -> [w734]
        tunnel: w713 -> [w733]
        tunnel: w712 -> [w729]
        shift-right: [w723] -> _
        shift-left: dbl[][] [] -> [w724]
        stop <- w758 stop-if-true
        n286 = First Call?() -> (First Call?: T/F=w740:bool)
        n287 = case shown="True" w740 {
          tunnel: w739 -> [w759 w764]
          tunnel: w738 -> [w760 w763]
          tunnel: [w759 w762] -> w737
          tunnel: [w760 w761] -> w736
          frame False {
          }
          frame True {
            n288 = call <vilib>:"DAQmx Start Task.vi"("task/channels in"=w764, "error in"=w763) -> ("task out"=w762:refnum<k21>, "error out"=w761:errorcluster)  [unwired: 12 in]
          }
        }
        n289 = local read "Pulser Cycles"() -> (w741:i32)
        n290 = call-poly <vilib>:"DAQmx Read.vi"("task/channels in"=w737, "number of samples per channel"=w729, "error in"=w736) -> ("task out"=w757:refnum<k21>, "data"=w727:waveform(dbl)[], "error out"=w756:errorcluster)  [unwired: 10 in]
        n291 = Quotient & Remainder(x=w742, y=w741) -> (x-y*floor(x/y)=w754:i32)  [unwired: 1 out]
        n292 = Equal To 0?(x=w754) -> (x = 0?=w732:bool)
        n293 = Index Array(array=w727, index #1=0 ("index (row)"), index #2=1 ("index")) -> (element #1=w730:waveform(dbl), element #2=w725:waveform(dbl))
        n294 = Unbundle By Name(w730) -> ("Y"=w728:dbl[])
        n295 = Add(x=w728, y=w753) -> (x+y=w750:dbl[])
        n296 = case shown="True" w732 {
          tunnel: w741 -> [_ w792]
          tunnel: w730 -> [_ w786]
          tunnel: w750 -> [w770 w798]
          tunnel: [w770 w797] -> w752
          tunnel: w751 -> [_ w797]
          tunnel: [w769 w795] -> w749
          tunnel: w748 -> [w769 w796]
          tunnel: w747 -> [_ w781]
          tunnel: [w768 w793] -> w746
          tunnel: w745 -> [w768 w794]
          tunnel: [w766 1 ("Average")] -> w743
          tunnel: w742 -> [w767 _]
          tunnel: w735 -> [_ w782]
          tunnel: w734 -> [_ w784]
          tunnel: w733 -> [_ w783]
          tunnel: w725 -> [_ _]
          tunnel: [w765 w773] -> w723
          tunnel: w724 -> [w765 w771]
          frame False {
            n297 = Increment(x=w767) -> (x+1=w766:i32)
          }
          frame True {
            n298 = Divide(x=w798, y=w792) -> (x/y=w772:dbl[])
            n299 = Bundle By Name(cluster=w786, "Y"=w772) -> (w787:waveform(dbl))
            n300 = xnode "Spectral Measurements"("신호"=w787) -> ("PSD"=w789:cluster{"f0":dbl, "df":dbl, "magnitude":dbl[]})  [unwired: 1 in, 1 out]
            n301 = call "PECT_Feature extraction.vi"("Length T/2"=w781, "Offset"="Offset", "Length"=w782, "Start 2"=w783, "Start 1"=w784, "Pulse signal in"=w772) -> ("Feature extraction out"=→"Feature Extraction":dbl)  [unwired: 5 in]
            n302 = case shown="True" "2 Plots" {
              tunnel: [w806 w812] -> w779
              tunnel: w796 -> [_ w811]
              tunnel: [w803 w811] -> w795
              tunnel: w787 -> [w803 w807]
              tunnel: w789 -> [w804 w809]
              tunnel: [w805 w810] -> w788
              tunnel: w794 -> [_ w808]
              tunnel: [w804 w808] -> w793
              frame False {
                n303 = Build Array(w804, w804) -> (w805:cluster{"f0":dbl, "df":dbl, "magnitude":dbl[]}[])
                n304 = Build Array(w803, w803) -> (w806:waveform(dbl)[])
              }
              frame True {
                n305 = Build Array(w808, w809) -> (w810:cluster{"f0":dbl, "df":dbl, "magnitude":dbl[]}[])
                n306 = Build Array(w811, w807) -> (w812:waveform(dbl)[])
              }
            }
            "Power spectral density" <- w788
            "Hall sensors signal" <- w779
            n307 = case shown="True" "Add LF" {
              tunnel: w772 -> [_ w802]
              tunnel: [w799 w800] -> w773
              tunnel: w771 -> [w799 w801]
              frame False {
              }
              frame True {
                n308 = Build Array (concatenate)(w801, w802) -> (w800:dbl[][])
              }
            }
            n309 = call "CSV Save.vi"("Array"=w773, "Save Button"="Save LF") -> ()  [unwired: 9 in, 1 out]
            n310 = Delete From Array(array=w773, index (col)=0 ("disabled index (col)")) -> (array with subset deleted=w774:dbl[][])  [unwired: 2 in, 1 out]
            n311 = Subtract(x=w774, y=w773) -> (x-y=→"dy":dbl[][])
          }
        }
        n312 = local read "Exit"() -> (w744:bool)
        n313 = Unbundle By Name(w756) -> ("status"=w755:bool)
        n314 = Or(x=w755, y=w744) -> (x .or. y?=w758:bool)
      }
    }
  }
  n315 = VISA Close(VISA resource name=w37, error in (no error)=w36) -> (error out=w34:errorcluster)
  n316 = VISA Close(VISA resource name=w38, error in (no error)=w39) -> (error out=w35:errorcluster)
  n317 = call <vilib>:"Simple Error Handler.vi"("error in (no error)"=w34) -> ()  [unwired: 4 in, 5 out]
  n318 = call <vilib>:"Simple Error Handler.vi"("error in (no error)"=w35) -> ()  [unwired: 4 in, 5 out]
  n319 = while {
    shift-right: [w842] -> _
    shift-left: T1."No Scan" -> [w847]
    shift-right: [w838] -> _
    shift-left: 0.0 ("Current  Position (mm)") -> [w846]
    shift-right: [w839] -> _
    shift-left: 0.0 ("Current  Position (mm)") -> [w845]
    shift-right: [w837] -> _
    shift-left: 0.0 ("Current  Position (mm)") -> [w844]
    shift-right: [w836] -> _
    shift-left: 0.0 ("Current  Position (mm)") -> [w843]
    tunnel: w24 -> [w841]
    tunnel: w23 -> [w828]
    tunnel: w26 -> [w840]
    tunnel: w25 -> [w827]
    tunnel: [w835] -> _
    tunnel: [w833] -> w32
    tunnel: [w834] -> _
    tunnel: [w832] -> w33
    shift-right: [w825] -> _
    shift-left: 0.0 ("Current  Position (mm)") -> [w824]
    stop <- w829 stop-if-true
    n320 = case shown="\"Wait X\"" w847 {
      selector: w847 -> [w866 _ _ _ _]
      tunnel: w846 -> [w859 w926 w948 w1012 w1052]
      tunnel: w845 -> [w860 w925 w954 w1011 w1051]
      tunnel: w844 -> [_ w924 w971 w992 w1035]
      tunnel: w843 -> [_ w923 w972 w1010 w1033]
      tunnel: [w865 T1."Wait X" w950 w1003 w1037] -> w842
      tunnel: w841 -> [w864 w918 w967 w1001 w1046]
      tunnel: w828 -> [w863 w919 w968 w1002 w1047]
      tunnel: w840 -> [w862 w920 w960 w997 w1049]
      tunnel: w827 -> [w861 w921 w961 w998 w1048]
      tunnel: [w852 w925 w954 w1011 w1051] -> w839
      tunnel: [w851 w926 w951 w1012 w1052] -> w838
      tunnel: [w854 w924 w971 w992 w1050] -> w837
      tunnel: [w853 w923 w972 w1010 w1033] -> w836
      tunnel: [w858 w912 w965 w1000 w1044] -> w835
      tunnel: [w857 w911 w963 w999 w1042] -> w833
      tunnel: [w856 w910 w969 w995 w1040] -> w834
      tunnel: [w855 w909 w970 w996 w1038] -> w832
      tunnel: w828 -> [_ _ _ _ _]
      tunnel: [w850 w908 w941 w990 w1029] -> w825
      tunnel: w824 -> [w849 w908 w947 w990 w1029]
      frame "No Scan", Default {
        n321 = local read "Scan"() -> (w848:bool)
        n322 = case shown="True" w848 {
          tunnel: w866 -> [w874 _]
          tunnel: [w874 w885] -> w865
          tunnel: w864 -> [w871 w883]
          tunnel: w863 -> [w872 w882]
          tunnel: w862 -> [w869 w881]
          tunnel: w861 -> [w870 w880]
          tunnel: w860 -> [w868 _]
          tunnel: w859 -> [w873 _]
          tunnel: [w873 w879] -> w851
          tunnel: [w872 w889] -> w858
          tunnel: [w871 w888] -> w857
          tunnel: [w870 w887] -> w856
          tunnel: [w869 w886] -> w855
          tunnel: [w868 w884] -> w854
          tunnel: [w867 w879] -> w850
          tunnel: w849 -> [w867 _]
          frame False {
          }
          frame True {
            n323 = flat-sequence {
              tunnel: w880 -> [w890]
              tunnel: w881 -> [w891]
              tunnel: w882 -> [w892]
              tunnel: w883 -> [w893]
              tunnel: [w893] -> w878
              tunnel: [w892] -> w877
              tunnel: [w891] -> w876
              tunnel: [w890] -> w875
              tunnel: [w907] -> w889
              tunnel: [w906] -> w888
              tunnel: [w905] -> w887
              tunnel: [w904] -> w886
              tunnel: [T1."Move X"] -> w885
              tunnel: [w902] -> w884
              tunnel: [w895] -> w879
              tunnel: w878 -> [w901]
              tunnel: w877 -> [w900]
              tunnel: w876 -> [w899]
              tunnel: w875 -> [w898]
              frame #0 {
              }
              frame #1 {
                n324 = local write "Direction (+)"("+" ("Direction (+)")) -> ()
                n325 = local write "Numeric"(0.0 ("Numeric")) -> ()
                n326 = local read "Travel per Pulse (mm)"() -> (w897:dbl)
                n327 = call "Autonics_GetPos.vi"("error in (no error)"=w901, "Travel per Pulse (mm)"=w897, "VISA resource name"=w900) -> ("error out"=w906:errorcluster, "Current  Position (mm)"=w895:dbl, "VISA resource name out"=w907:refnum<visa-resource-name>)  [unwired: 6 in]
                "Start Pos Y" <- w895
                n328 = call "Autonics_GetPos.vi"("error in (no error)"=w899, "Travel per Pulse (mm)"=w897, "VISA resource name"=w898) -> ("error out"=w904:errorcluster, "Current  Position (mm)"=w902:dbl, "VISA resource name out"=w905:refnum<visa-resource-name>)  [unwired: 6 in]
                "Start Pos X" <- w902
                n329 = local write "Cur. Pos X"(w895) -> ()
                n330 = local write "Cur. Pos Y"(w902) -> ()
              }
            }
          }
        }
        n331 = local read "X - length"() -> (w852:dbl)
        n332 = local read "Step Y"() -> (w853:dbl)
      }
      frame "Move X" {
        n333 = local read "Travel per Pulse (mm)"() -> (w913:dbl)
        n334 = local read "X - length"() -> (w914:dbl)
        n335 = call "Autonics_Move.vi"("Direction (+)"="Direction (+)", "error in (no error)"=w918, "Travel per Pulse (mm)"=w913, "Move Distance (mm)"=w914, "VISA resource name"=w919) -> ("error out"=w916:errorcluster, "VISA resource name out"=w917:refnum<visa-resource-name>)  [unwired: 5 in]
        n336 = flat-sequence {
          tunnel: [w931] -> w912
          tunnel: w917 -> [w931]
          tunnel: [w930] -> w911
          tunnel: w916 -> [w930]
          tunnel: [w928] -> w910
          tunnel: w921 -> [w928]
          tunnel: [w927] -> w909
          tunnel: w920 -> [w927]
          frame #0 {
            n337 = Wait (ms)(milliseconds to wait=u32 100) -> ()  [unwired: 1 out]
          }
        }
      }
      frame "Wait X" {
        n338 = local read "Travel per Pulse (mm)"() -> (w958:dbl)
        n339 = call "Autonics_GetPos.vi"("error in (no error)"=w960, "Travel per Pulse (mm)"=w958, "VISA resource name"=w961) -> ("error out"=w959:errorcluster, "Current  Position (mm)"=w957:dbl, "VISA resource name out"=w962:refnum<visa-resource-name>)  [unwired: 6 in]
        n340 = call "Autonics_GetPos.vi"("error in (no error)"=w967, "Travel per Pulse (mm)"=w958, "VISA resource name"=w968) -> ("error out"=w964:errorcluster, "Current  Position (mm)"=w939:dbl, "VISA resource name out"=w966:refnum<visa-resource-name>)  [unwired: 6 in]
        n341 = local read "Direction (+)"() -> (w934:string)
        n342 = local write "Cur. Pos Y"(w957) -> ()
        n343 = Equal?(x=w934, y="-") -> (x = y?=w932:bool)
        n344 = local read "Step X"() -> (w944:dbl)
        n345 = local write "Cur. Pos X"(w939) -> ()
        n346 = Subtract(x=w939, y=w947) -> (x-y=w946:dbl)
        n347 = Absolute Value(x=w954) -> (abs(x)=w956:dbl)
        n348 = Absolute Value(x=w946) -> (abs(x)=w945:dbl)
        n349 = Subtract(x=w939, y=w948) -> (x-y=w955:dbl)
        n350 = Greater Or Equal?(x=w945, y=w944) -> (x >= y?=w940:bool)
        n351 = Quotient & Remainder(x=w939, y=w944) -> (floor(x/y)=w936:dbl)  [unwired: 1 out]
        n352 = Absolute Value(x=w955) -> (abs(x)=w949:dbl)
        n353 = Subtract(x=w949, y=w956) -> (x-y=w952:dbl)
        n354 = case shown="True" w940 {
          selector: w940 -> [_ w973]
          frame False {
          }
          frame True {
            n355 = local read "Numeric"() -> (w975:dbl)
            n356 = Increment(x=w975) -> (x+1=→"Numeric":dbl)
            "Acquire" <- w973
          }
        }
        n357 = Increment(x=w936) -> (x+1=w937:dbl)
        n358 = call "Convert Double Precision.vi"("Input"=w952) -> ("Output"=w953:dbl)  [unwired: 10 in]
        n359 = Select(t=w937, s=w932, f=w936) -> (s? t:f=w935:dbl)
        n360 = Multiply(x=w935, y=w944) -> (x*y=w943:dbl)
        n361 = Select(t=w943, s=w940, f=w947) -> (s? t:f=w942:dbl)
        n362 = Greater Or Equal To 0?(x=w953) -> (x >= 0?=w938:bool)
        n363 = Select(t=w939, s=w938, f=w942) -> (s? t:f=w941:dbl)
        n364 = case shown="True" w938 {
          tunnel: [w978 w989] -> w970
          tunnel: w959 -> [w978 w989]
          tunnel: [w979 w988] -> w969
          tunnel: w962 -> [w979 w988]
          tunnel: [w981 w987] -> w965
          tunnel: w966 -> [w981 w987]
          tunnel: [w980 w986] -> w963
          tunnel: w964 -> [w980 w986]
          tunnel: [w977 w985] -> w951
          tunnel: w948 -> [w977 _]
          tunnel: [T1."Wait X" T1."Move Y"] -> w950
          frame False {
          }
          frame True {
            n365 = local read "Cur. Pos X"() -> (w985:dbl)
            n366 = local write "Numeric"(0.0 ("Numeric")) -> ()
            n367 = Wait (ms)(milliseconds to wait=u32 1000) -> ()  [unwired: 1 out]
          }
        }
        "Current  Position (mm)" <- w947
      }
      frame "Move Y" {
        n368 = local read "Step Y"() -> (w1006:dbl)
        n369 = local read "Y - length"() -> (w991:dbl)
        n370 = local read "Start Pos Y"() -> (w993:dbl)
        n371 = Subtract(x=w991, y=w1006) -> ()  [unwired: 1 out]
        n372 = Subtract(x=w993, y=w992) -> (x-y=w1009:dbl)
        n373 = Absolute Value(x=w991) -> (abs(x)=w1007:dbl)
        n374 = Absolute Value(x=w1009) -> (abs(x)=w1008:dbl)
        n375 = Subtract(x=w1008, y=w1007) -> (x-y=w1005:dbl)
        n376 = call "Convert Double Precision.vi"("Input"=w1005) -> ("Output"=w1004:dbl)  [unwired: 10 in]
        n377 = Greater Or Equal To 0?(x=w1004) -> (x >= 0?=w994:bool)
        n378 = case shown="True" w994 {
          tunnel: [T1."Wait Y" T1."No Scan"] -> w1003
          tunnel: w1002 -> [w1020 w1026]
          tunnel: [w1021 w1025] -> w999
          tunnel: w1001 -> [w1021 w1025]
          tunnel: [w1020 w1026] -> w1000
          tunnel: w998 -> [w1014 w1024]
          tunnel: w997 -> [w1018 w1023]
          tunnel: [w1019 w1023] -> w996
          tunnel: [w1013 w1024] -> w995
          frame False {
            n379 = local read "Step Y"() -> (w1017:dbl)
            n380 = local read "Travel per Pulse (mm)"() -> (w1015:dbl)
            n381 = call "Autonics_Move.vi"("Direction (+)"="+" ("Direction (+) 2"), "error in (no error)"=w1018, "Travel per Pulse (mm)"=w1015, "Move Distance (mm)"=w1017, "VISA resource name"=w1014) -> ("error out"=w1019:errorcluster, "VISA resource name out"=w1013:refnum<visa-resource-name>)  [unwired: 5 in]
          }
          frame True {
            n382 = local write "Scan"(FALSE) -> ()
          }
        }
      }
      frame "Wait Y" {
        n383 = local read "Travel per Pulse (mm)"() -> (w1030:dbl)
        n384 = call "Autonics_GetPos.vi"("error in (no error)"=w1049, "Travel per Pulse (mm)"=w1030, "VISA resource name"=w1048) -> ("error out"=w1039:errorcluster, "Current  Position (mm)"=w1034:dbl, "VISA resource name out"=w1041:refnum<visa-resource-name>)  [unwired: 6 in]
        n385 = call "Autonics_GetPos.vi"("error in (no error)"=w1046, "Travel per Pulse (mm)"=w1030, "VISA resource name"=w1047) -> ("error out"=w1043:errorcluster, "Current  Position (mm)"=w1036:dbl, "VISA resource name out"=w1045:refnum<visa-resource-name>)  [unwired: 6 in]
        n386 = Subtract(x=w1034, y=w1035) -> (x-y=w1054:dbl)
        n387 = Absolute Value(x=w1033) -> (abs(x)=w1056:dbl)
        n388 = Absolute Value(x=w1054) -> (abs(x)=w1055:dbl)
        n389 = Subtract(x=w1055, y=w1056) -> (x-y=w1053:dbl)
        n390 = local write "Cur. Pos X"(w1036) -> ()
        n391 = local write "Cur. Pos Y"(w1034) -> ()
        n392 = call "Convert Double Precision.vi"("Input"=w1053) -> ("Output"=w1032:dbl)  [unwired: 10 in]
        n393 = Greater Or Equal To 0?(x=w1032) -> (x >= 0?=w1031:bool)
        n394 = case shown="True" w1031 {
          tunnel: w1035 -> [w1062 _]
          tunnel: [w1062 w1075] -> w1050
          tunnel: w1045 -> [w1061 w1073]
          tunnel: [w1061 w1073] -> w1044
          tunnel: [w1060 w1072] -> w1042
          tunnel: w1043 -> [w1060 w1072]
          tunnel: [w1059 w1071] -> w1040
          tunnel: w1041 -> [w1059 w1071]
          tunnel: [w1058 w1070] -> w1038
          tunnel: w1039 -> [w1058 w1070]
          tunnel: [T1."Wait Y" T1."Move X"] -> w1037
          frame False {
          }
          frame True {
            n395 = local read "Direction (+)"() -> (w1069:string)
            n396 = local read "Cur. Pos Y"() -> (w1075:dbl)
            n397 = Equal?(x=w1069, y="+") -> (x = y?=w1067:bool)
            n398 = Select(t="-", s=w1067, f="+") -> (s? t:f=w1066:string)
            n399 = local write "Direction (+)"(w1066) -> ()
            n400 = Wait (ms)(milliseconds to wait=u32 1000) -> ()  [unwired: 1 out]
          }
        }
      }
    }
    n401 = Wait Until Next ms Multiple(millisecond multiple=u32 100 ("milliseconds to wait")) -> ()  [unwired: 1 out]
    n402 = local read "Completed"() -> (w823:bool)
    n403 = local read "Exit"() -> (w822:bool)
    n404 = Unbundle By Name(w832) -> ("status"=w830:bool)
    n405 = Unbundle By Name(w833) -> ("status"=w831:bool)
    n406 = Compound Arithmetic op=OR(w823, w822, w831, w830) -> (w829:bool)
    "Enum" <- w847
  }
  n407 = call <vilib>:"DAQmx Clear Task.vi"("task in"=w89, "error in"=w88) -> ("error out"=w95:errorcluster)  [unwired: 13 in]
  n408 = call <vilib>:"Simple Error Handler.vi"("error in (no error)"=w95) -> ()  [unwired: 4 in, 5 out]
  n409 = call <vilib>:"Simple Error Handler.vi"("error in (no error)"=w32) -> ()  [unwired: 4 in, 5 out]
  n410 = call <vilib>:"Simple Error Handler.vi"("error in (no error)"=w33) -> ()  [unwired: 4 in, 5 out]
  n411 = call <vilib>:"Simple Error Handler.vi"() -> ()  [unwired: 5 in, 5 out]
